vi "single fit V5cpp.vi"(0 "single fit parameters":T11={"number of 2D grid points"=300, "# of points in pond"=339, "# of points in window"=10919, "decimation threshold"=1, "normalization factor"=0.029014793, "pond scale factor "=3.0, "normalized z"=[], "decimated z"=[], "decimated omega"=[], "omega in window"=[], "z in window"=[], "data center"=3.0+0.0i, "inverse"=[], "linear "=[], "omega around"=[], "phase around center"=[], "fit for phase around senter "=[], "three points"={[], []}, "max omega"=0.029014793, "min omega"=0.029014793, "dz/domega"=[]}, 1 "plot what":enum16{"plot", "dont plot", "a"}(ring), 2 "find fit action":T8=enum."bbb", 3 "cursor bracket: fragment  ref":refnum<vi>, 5 "omega map parameters":T10={"map method"=enum."less trivial", "2:window factor"=1, "left"=3.0, "right"=3.0, "omega"=3.0, "gamma"=3.0, "theta0"=3.0, "use points"=enum."decimated", "z(inf) method"=enum."median"}, 7 "parameters: wavepacket":T4={"R"=0.5, "wave number"=9.317073170731707, "delta k"=8.0, "radii vector"=[-1.5, -1.4361702127659575, -1.372340425531915, -1.3085106382978724, -1.2446808510638299, -1.1808510638297873, -1.1170212765957448, -1.0531914893617023, -0.9893617021276596, -0.9255319148936171, -0.8617021276595745, -0.797872340425532, -0.7340425531914894, -0.6702127659574468, -0.6063829787234043, -0.5425531914893618, -0.47872340425531923, -0.4148936170212767, -0.35106382978723416, -0.2872340425531916, -0.2234042553191491, -0.15957446808510656, -0.09574468085106402, -0.03191489361702149, 0.03191489361702127, 0.0957446808510638, 0.15957446808510634, 0.22340425531914887, 0.2872340425531914, 0.35106382978723394, 0.4148936170212765, 0.478723404255319, 0.5425531914893615, 0.6063829787234041, 0.6702127659574466, 0.7340425531914891, 0.7978723404255317, 0.8617021276595742, 0.9255319148936167, 0.9893617021276593, 1.0531914893617018, 1.1170212765957444, 1.1808510638297869, 1.2446808510638294, 1.308510638297872, 1.3723404255319145, 1.436170212765957], "radial section"=[-0.0004435445083409722-0.0006849119769038184i, -0.0019041504025470312+0.00048506615579312746i, -0.00033819317362592454+0.00445256884703147i, 0.008816469374270853+0.0037385059601190047i, 0.012871051762105094-0.014489928742809924i, -0.018368300887416027-0.03213667871181133i, -0.06546452421830008+0.012862287260149104i, -0.014850036489490822+0.11250194158627941i, 0.16349796399613198+0.08029027224632529i, 0.19438455385148304-0.19581588584379236i, -0.1764517694229995-0.3527505964833319i, -0.5269831636950821+0.07349813170268539i, -0.12571385568454752+0.6656158756342778i, 0.7094879059571741+0.3986438774133789i, 0.6853115356988965-0.6177994674685856i, -0.39205198313530026-0.9060192033187687i, -0.9933425353192824+0.08278273424671147i, -0.22770617853759392+0.9220982637950581i, 0.720265950295077+0.4589746661280373i, 0.564369978321562-0.45471185099562045i, -0.20063123992670956-0.5446207511436068i, -0.438459632746935+0.012155082564416607i, -0.0917074180027409+0.299079584121901i, 0.17101533661135507+0.12280738192151135i, 0.17101533661135532+0.1228073819215104i, -0.0917074180027395+0.299079584121901i, -0.4384596327469345+0.01215508256441854i, -0.2006312399267118-0.5446207511436055i, 0.5643699783215596-0.4547118509956226i, 0.7202659502950789+0.45897466612803384i, -0.22770617853759056+0.9220982637950585i, -0.9933425353192818+0.08278273424671675i, -0.3920519831353035-0.9060192033187675i, 0.6853115356988935-0.6177994674685894i, 0.7094879059571758+0.3986438774133766i, -0.12571385568454407+0.665615875634279i, -0.5269831636950825+0.0734981317026883i, -0.17645176942300106-0.3527505964833319i, 0.19438455385148207-0.19581588584379414i, 0.16349796399613292+0.0802902722463243i, -0.014850036489490074+0.11250194158627992i, -0.06546452421830022+0.012862287260149614i, -0.018368300887416446-0.032136678711811265i, 0.012871051762104992-0.014489928742810118i, 0.008816469374270927+0.0037385059601189627i, -0.0003381931736258947+0.004452568847031496i, -0.0019041504025470377+0.00048506615579315077i], "wave vector"=19.513632417419526, "wavepacket is"=TRUE} {"delta k" format="%#_3f"; "wave number" format="%#_3f"; "R" format="%#_3f"}, 9 "parameters: complex fit":T3={"main VI path"=path "", "scale factor"=3.0, "# of grid points"=200, "parameters: wavepacket"={"R"=0.5, "wave number"=22.0, "delta k"=7.0, "radii vector"=[], "radial section"=[], "wave vector"=22.0, "wavepacket is"=TRUE}, "span"=0.27789, "interference ?"=enum."cp z center", "filter method"=enum."three"} {"span" min=0.0 max=0.5 step=1e-05 scale=0.0001..0.5 scale format="%#_5f"; "parameters: wavepacket"."delta k" format="%#_3f"; "parameters: wavepacket"."wave number" format="%#_3f"; "parameters: wavepacket"."R" format="%#_3f"}, 11 "input":cdb, 13 "plots: filter related":T6) -> (4 "single fit parameters out":T11={"number of 2D grid points"=300, "# of points in pond"=339, "# of points in window"=10919, "decimation threshold"=1, "normalization factor"=0.029014793, "pond scale factor "=3.0, "normalized z"=[], "decimated z"=[], "decimated omega"=[], "omega in window"=[], "z in window"=[], "data center"=3.0+0.0i, "inverse"=[], "linear "=[], "omega around"=[], "phase around center"=[], "fit for phase around senter "=[], "three points"={[], []}, "max omega"=0.029014793, "min omega"=0.029014793, "dz/domega"=[]}, 6 "omega map parameters out":T10={"map method"=enum."less trivial", "2:window factor"=1, "left"=3.0, "right"=3.0, "omega"=3.0, "gamma"=3.0, "theta0"=3.0, "use points"=enum."decimated", "z(inf) method"=enum."median"}, 8 "parameters: wavepacket  out":T4={"R"=0.5, "wave number"=9.317073170731707, "delta k"=8.0, "radii vector"=[-1.5, -1.4361702127659575, -1.372340425531915, -1.3085106382978724, -1.2446808510638299, -1.1808510638297873, -1.1170212765957448, -1.0531914893617023, -0.9893617021276596, -0.9255319148936171, -0.8617021276595745, -0.797872340425532, -0.7340425531914894, -0.6702127659574468, -0.6063829787234043, -0.5425531914893618, -0.47872340425531923, -0.4148936170212767, -0.35106382978723416, -0.2872340425531916, -0.2234042553191491, -0.15957446808510656, -0.09574468085106402, -0.03191489361702149, 0.03191489361702127, 0.0957446808510638, 0.15957446808510634, 0.22340425531914887, 0.2872340425531914, 0.35106382978723394, 0.4148936170212765, 0.478723404255319, 0.5425531914893615, 0.6063829787234041, 0.6702127659574466, 0.7340425531914891, 0.7978723404255317, 0.8617021276595742, 0.9255319148936167, 0.9893617021276593, 1.0531914893617018, 1.1170212765957444, 1.1808510638297869, 1.2446808510638294, 1.308510638297872, 1.3723404255319145, 1.436170212765957], "radial section"=[-0.0004435445083409722-0.0006849119769038184i, -0.0019041504025470312+0.00048506615579312746i, -0.00033819317362592454+0.00445256884703147i, 0.008816469374270853+0.0037385059601190047i, 0.012871051762105094-0.014489928742809924i, -0.018368300887416027-0.03213667871181133i, -0.06546452421830008+0.012862287260149104i, -0.014850036489490822+0.11250194158627941i, 0.16349796399613198+0.08029027224632529i, 0.19438455385148304-0.19581588584379236i, -0.1764517694229995-0.3527505964833319i, -0.5269831636950821+0.07349813170268539i, -0.12571385568454752+0.6656158756342778i, 0.7094879059571741+0.3986438774133789i, 0.6853115356988965-0.6177994674685856i, -0.39205198313530026-0.9060192033187687i, -0.9933425353192824+0.08278273424671147i, -0.22770617853759392+0.9220982637950581i, 0.720265950295077+0.4589746661280373i, 0.564369978321562-0.45471185099562045i, -0.20063123992670956-0.5446207511436068i, -0.438459632746935+0.012155082564416607i, -0.0917074180027409+0.299079584121901i, 0.17101533661135507+0.12280738192151135i, 0.17101533661135532+0.1228073819215104i, -0.0917074180027395+0.299079584121901i, -0.4384596327469345+0.01215508256441854i, -0.2006312399267118-0.5446207511436055i, 0.5643699783215596-0.4547118509956226i, 0.7202659502950789+0.45897466612803384i, -0.22770617853759056+0.9220982637950585i, -0.9933425353192818+0.08278273424671675i, -0.3920519831353035-0.9060192033187675i, 0.6853115356988935-0.6177994674685894i, 0.7094879059571758+0.3986438774133766i, -0.12571385568454407+0.665615875634279i, -0.5269831636950825+0.0734981317026883i, -0.17645176942300106-0.3527505964833319i, 0.19438455385148207-0.19581588584379414i, 0.16349796399613292+0.0802902722463243i, -0.014850036489490074+0.11250194158627992i, -0.06546452421830022+0.012862287260149614i, -0.018368300887416446-0.032136678711811265i, 0.012871051762104992-0.014489928742810118i, 0.008816469374270927+0.0037385059601189627i, -0.0003381931736258947+0.004452568847031496i, -0.0019041504025470377+0.00048506615579315077i], "wave vector"=19.513632417419526, "wavepacket is"=TRUE} {"delta k" format="%#_3f"; "wave number" format="%#_3f"; "R" format="%#_3f"}, 14 "complex region out":T7={"max re"=1.1965102077412717, "min re"=-1.8034897922587283, "max im"=1.1920568931854867, "min im"=-1.636084117505164, "delta re"=3.0, "delta im"=2.8281410106906506, "center re"=-0.3034897922587282, "delta  z"=3.0+2.8281410106906506i, "center im"=-0.2220136121598386, "center z"=-0.3034897922587282+2.8281410106906506i, "d im"=0.0, "d re"=0.0, "d z"=0.0+0.0i}, 15 "lorentzian out":T1={"A (VHz)"=-1.0311345636926572, "ω (Hz)"=-1.0311345636926572, "Γ (Hz)"=-1.0311345636926572, "φ (rad)"=-1.0311345636926572, "Q"=-1.0311345636926572, "Norm  Ampl"=-1.0311345636926572, "z∞ (V)"=-1.0311345636926572+0.0i, "4corners"={"z (-pi/2)"=-1.0311345636926572+0.5736824521422934i, "z(inf)"=-0.5200164984937075+1.0975277942502903i, "z (pi/2)"=-1.0311345636926572+0.5736824521422934i, "z center"=-0.5136528600391839+0.580046090596817i, "z(0)"=-0.5200164984937075+1.0975277942502903i, "radius"=-1.0311345636926572}} {"z∞ (V)" format="%#_4p"; "Q" format="%#_4p"; "φ (rad)" format="%#_3p"; "Γ (Hz)" format="%#_5p"; "ω (Hz)" format="%#_9p"; "A (VHz)" format="%#_3p"})   [LabVIEW 2021]
uses:
  circle corners.ctl
  lorentzian.ctl
  find peak action.ctl
  stack action -- control.ctl
  cursor window action.ctl
  circledll.dll
  complex region.ctl
  single fit parameters.ctl
  omega map parameters.ctl
  cursor winow.ctl
  wavepacket.ctl
  plot refs -- filter related.ctl
  filter method control.ctl
  peak -- parameters -- complex fit.ctl
panel:
  out "counter_out":i32
  out "# points in window":dbl
  out "good lorentzian":T1={"A (VHz)"=-1.0311345636926572, "ω (Hz)"=-1.0311345636926572, "Γ (Hz)"=-1.0311345636926572, "φ (rad)"=-1.0311345636926572, "Q"=-1.0311345636926572, "Norm  Ampl"=-1.0311345636926572, "z∞ (V)"=-1.0311345636926572+0.0i, "4corners"={"z (-pi/2)"=-1.0311345636926572+0.5736824521422934i, "z(inf)"=-0.5200164984937075+1.0975277942502903i, "z (pi/2)"=-1.0311345636926572+0.5736824521422934i, "z center"=-0.5136528600391839+0.580046090596817i, "z(0)"=-0.5200164984937075+1.0975277942502903i, "radius"=-1.0311345636926572}} {"z∞ (V)" format="%#_4p"; "Q" format="%#_4p"; "φ (rad)" format="%#_3p"; "Γ (Hz)" format="%#_5p"; "ω (Hz)" format="%#_9p"; "A (VHz)" format="%#_3p"}
  out "cp lorentzian":T1={"A (VHz)"=-1.0311345636926572, "ω (Hz)"=-1.0311345636926572, "Γ (Hz)"=-1.0311345636926572, "φ (rad)"=-1.0311345636926572, "Q"=-1.0311345636926572, "Norm  Ampl"=-1.0311345636926572, "z∞ (V)"=-1.0311345636926572+0.0i, "4corners"={"z (-pi/2)"=-1.0311345636926572+0.5736824521422934i, "z(inf)"=-0.5200164984937075+1.0975277942502903i, "z (pi/2)"=-1.0311345636926572+0.5736824521422934i, "z center"=-0.5136528600391839+0.580046090596817i, "z(0)"=-0.5200164984937075+1.0975277942502903i, "radius"=-1.0311345636926572}} {"z∞ (V)" format="%#_4p"; "Q" format="%#_4p"; "φ (rad)" format="%#_3p"; "Γ (Hz)" format="%#_5p"; "ω (Hz)" format="%#_9p"; "A (VHz)" format="%#_3p"}
  out "pm lorentzian":T1={"A (VHz)"=-1.0311345636926572, "ω (Hz)"=-1.0311345636926572, "Γ (Hz)"=-1.0311345636926572, "φ (rad)"=-1.0311345636926572, "Q"=-1.0311345636926572, "Norm  Ampl"=-1.0311345636926572, "z∞ (V)"=-1.0311345636926572+0.0i, "4corners"={"z (-pi/2)"=-1.0311345636926572+0.5736824521422934i, "z(inf)"=-0.5200164984937075+1.0975277942502903i, "z (pi/2)"=-1.0311345636926572+0.5736824521422934i, "z center"=-0.5136528600391839+0.580046090596817i, "z(0)"=-0.5200164984937075+1.0975277942502903i, "radius"=-1.0311345636926572}} {"z∞ (V)" format="%#_4p"; "Q" format="%#_4p"; "φ (rad)" format="%#_3p"; "Γ (Hz)" format="%#_5p"; "ω (Hz)" format="%#_9p"; "A (VHz)" format="%#_3p"}
  in  "window factor - max":i32=10
  in  "window factor - min":i32=10
  out "bb 2":dbl
  out "directed sigma 2":dbl
  out "right 2":cdb
  out "left 2":cdb
  out "Numeric 2":i32
  in  "averaging -- win 2":dbl=1.3
  in  "averaging -- span 2":dbl=0.2
  in  "averaging -- # points 2":i32=30
  in  "averaging -- # points":i32=30
  in  "averaging -- span":dbl=0.2
  in  "averaging -- win":dbl=1.3
  out "Numeric":i32
  out "left":cdb
  out "right":cdb
  out "directed sigma":dbl
  out "bb":dbl
  in  "complex region":T7={"max re"=1.1965102077412717, "min re"=-1.8034897922587283, "max im"=1.1920568931854867, "min im"=-1.636084117505164, "delta re"=3.0, "delta im"=2.8281410106906506, "center re"=-0.3034897922587282, "delta  z"=3.0+2.8281410106906506i, "center im"=-0.2220136121598386, "center z"=-0.3034897922587282+2.8281410106906506i, "d im"=0.0, "d re"=0.0, "d z"=0.0+0.0i}
  in  "cursor bracket in":T9={"left"=2044.0881763527054, "right "=2126.7657992565055, "center"=2085.4269878046052, "window"=82.67762290380006, "cursors"=[], "relative"=0, "absolute"=0, "fixed vertical offset"=2421.6740576496672, "vertical offset"=2421.6740576496672, "skew"=2421.6740576496672, "default window frac"=2421.6740576496672, "kind"=enum."fancy", "skew.left"=2.0, "skew.right"=0.0, "Plot ref"=refnum, "wing order"=enum."back"}
  in  "factor":dbl=7.0
  in  "pond":cdb[][](array[numeric])
  in  "wave packet":cdb[][](array[numeric])
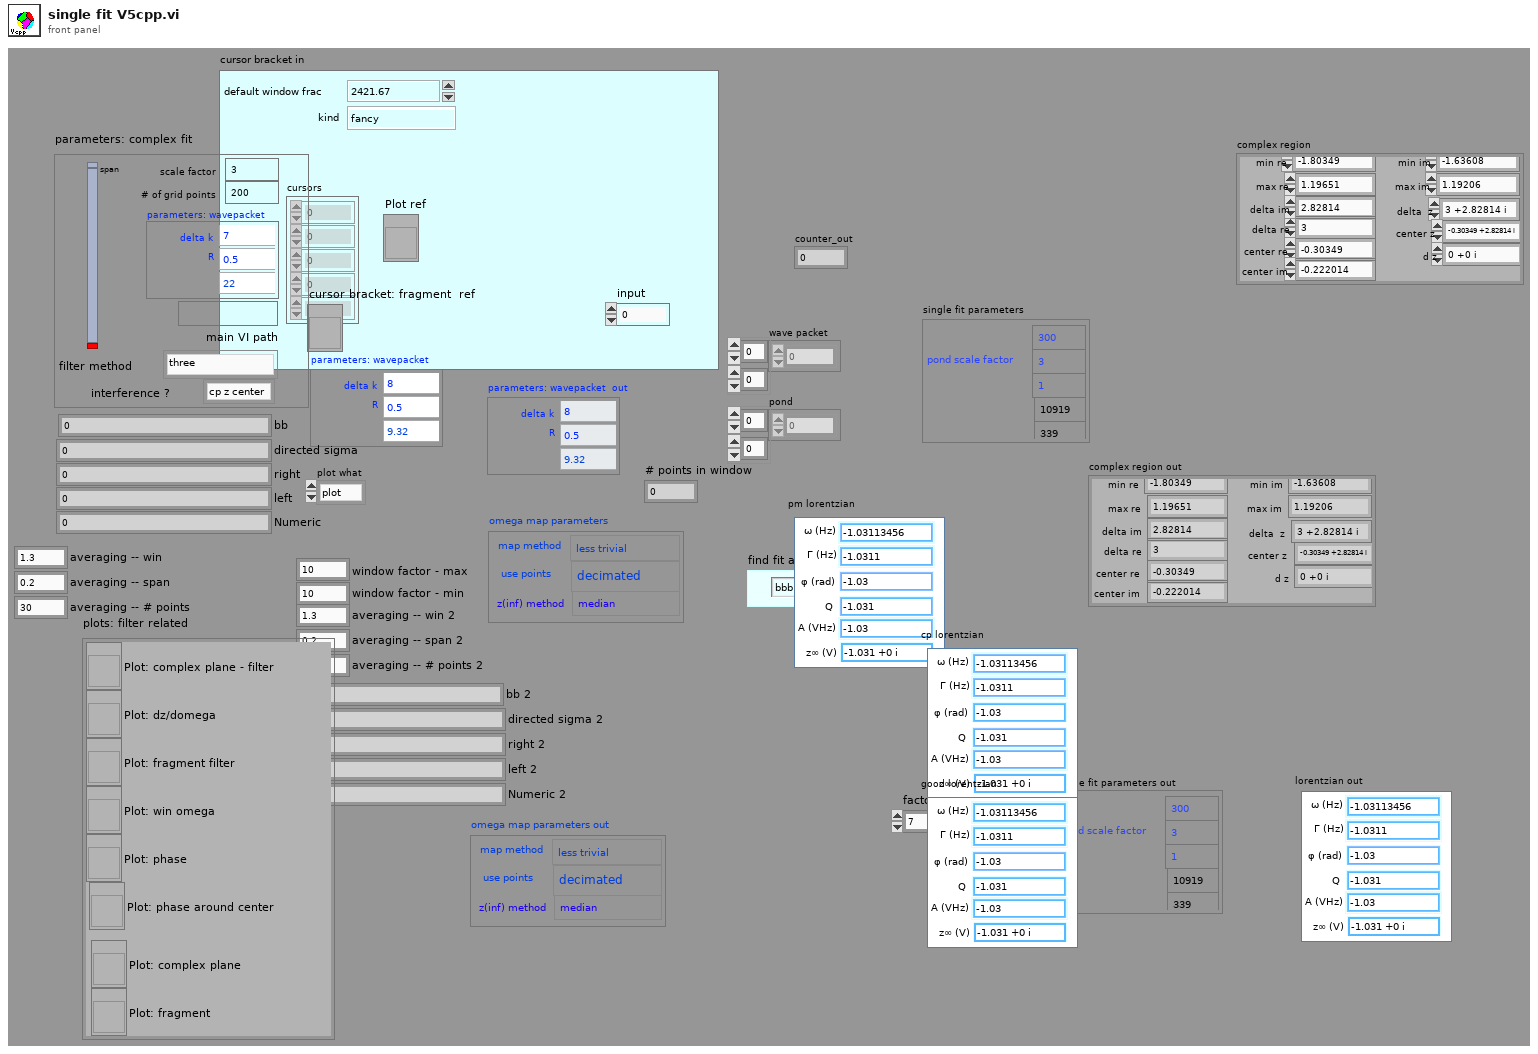
[diagram p1: front panel]
types:
  T1 = typedef "lorentzian.ctl" = cluster{"A (VHz)":dbl, "ω (Hz)":dbl, "Γ (Hz)":dbl, "φ (rad)":dbl, "Q":dbl, "Norm  Ampl":dbl, "z∞ (V)":cdb, "4corners":T2}
  T2 = typedef "circle corners.ctl" = cluster{"z (-pi/2)":cdb, "z(inf)":cdb, "z (pi/2)":cdb, "z center":cdb, "z(0)":cdb, "radius":dbl}
  T3 = typedef "peak -- parameters -- complex fit.ctl" = cluster{"main VI path":path, "scale factor":dbl, "# of grid points":i32, "parameters: wavepacket":T4, "span":dbl, "interference ?":enum16{"cp z center", "pm zcenter", "fancy"}, "filter method":T5}
  T4 = typedef "wavepacket.ctl" = cluster{"R":dbl, "wave number":dbl, "delta k":dbl, "radii vector":dbl[], "radial section":cdb[], "wave vector":dbl, "wavepacket is":bool}
  T5 = typedef "filter method control.ctl" = enum16{"four", "five", "one", "two", "three", "zero", "minus one", "minus two"}
  T6 = typedef "plot refs -- filter related.ctl" = cluster{"Plot: complex plane - filter":refnum<vi>, "Plot: dz/domega":refnum<vi>, "Plot: fragment filter":refnum<vi>, "Plot: win omega":refnum<vi>, "Plot: phase":refnum<vi>, "Plot: phase around center":refnum<vi>, "Plot: complex plane":refnum<vi>, "Plot: fragment":refnum<vi>}
  T7 = typedef "complex region.ctl" = cluster{"max re":dbl, "min re":dbl, "max im":dbl, "min im":dbl, "delta re":dbl, "delta im":dbl, "center re":dbl, "delta  z":cdb, "center im":dbl, "center z":cdb, "d im":dbl, "d re":dbl, "d z":cdb}
  T8 = typedef "find peak action.ctl" = enum16{"empty", "-find center", "-mapping", "fit", "-shake it one", "bbb", "-update pond", "move z(center)", "move z(inf)", "update pond", "fancy fit one", "fragment window moves", "-shake it two", "fancy fit two", "pm fit"}
  T9 = typedef "cursor winow.ctl" = cluster{"left":dbl, "right ":dbl, "center":dbl, "window":dbl, "cursors":i32[], "relative":i32, "absolute":i32, "fixed vertical offset":dbl, "vertical offset":dbl, "skew":dbl, "default window frac":dbl, "kind":enum16{"symmetric", "skewed", "fancy"}, "skew.left":dbl, "skew.right":dbl, "Plot ref":refnum<vi>, "wing order":enum16{"forw", "back"}}
  T10 = typedef "omega map parameters.ctl" = cluster{"map method":enum16{"simple", "less trivial", "around center", "geometry"}, "2:window factor":i32, "left":dbl, "right":dbl, "omega":dbl, "gamma":dbl, "theta0":dbl, "use points":enum16{"all in window", "decimated"}, "z(inf) method":enum16{"median", "method 2", "histogram"}}
  T11 = typedef "single fit parameters.ctl" = cluster{"number of 2D grid points":i32, "# of points in pond":i32, "# of points in window":i32, "decimation threshold":i32, "normalization factor":dbl, "pond scale factor ":dbl, "normalized z":cdb[], "decimated z":cdb[], "decimated omega":dbl[], "omega in window":dbl[], "z in window":cdb[], "data center":cdb, "inverse":cdb[], "linear ":cdb[], "omega around":dbl[], "phase around center":dbl[], "fit for phase around senter ":dbl[], "three points":cluster{dbl[], dbl[]}, "max omega":dbl, "min omega":dbl, "dz/domega":cdb[]}
  T12 = cluster{"cursor bracket: fragment  ref":refnum<vi>, "main VI path":path, "fancy fit":cluster{"z(center)":cdb, "center":dbl, "window":dbl, "omega ave":dbl, "gamma ave":dbl, "shakeit counter":i32, "current center":dbl, "current window":dbl}}
  T13 = typedef "stack action -- control.ctl" = enum16{"push", "pop", "check", "init"}
  T14 = typedef "cursor window action.ctl" = enum16{"balance", "h. offset change", "cursor moves", "change center", "change window", "init", "check", "reset", "set y to middle", "idle", "-write all Y", "-write left.X", "-write center.X", "-write right.X", "-write all X", "-change center", "-change window", "-change skew", "-read cursor 2", "-read cursor 1", "-read cursor 0", "-read all cursors", "-reset", "-read plot scale", "-set y to middle", "-Q: center.Y is visible", "-Q: window is visible", "-parse center.Y", "-right left from center", "-left move", "-right move", "-set center.Y", "-empty", "-set cursors to default", "-check", "-write center.Y", "-copy cursor 1", "-copy cursor 0", "-copy cursor 2", "move right", "move left", "shrink", "broaden", "skew up", "skew down", "-write plot scale", "zoom X", "change cen&win", "zoom to all data", "color--red", "color--green", "color--yellow", "read", "zoom out", "zoom in", "slide right", "slide left", "set range aspect ratio to 1", "move to window range", "--move to window range"}
  T15 = typedef "comparison control.ctl" = enum16{"not a number", "above", "in range", "below"}
  T16 = cluster{"left":dbl, "right ":dbl, "center":dbl, "window":dbl, "cursors":i32[], "relative":i32, "absolute":i32, "fixed vertical offset":dbl, "vertical offset":dbl, "skew":dbl, "default window frac":dbl, "kind":enum16{"symmetric", "skewed", "fancy"}, "skew.left":dbl, "skew.right":dbl, "Plot ref":refnum<vi>, "wing order":enum16{"forw", "back"}}
  T17 = enum16{"replace z(center) -- keepin z(inf) the same", "replace z(inf)  -- keeping z(center) the same"}
  T18 = typedef "tale of three indices -- int -- control.ctl" = cluster{"left":i32, "center":i32, "right":i32, "right most":i32, "left most":i32, "window":i32, "max win factor":i32, "max win":i32, "min win":i32}
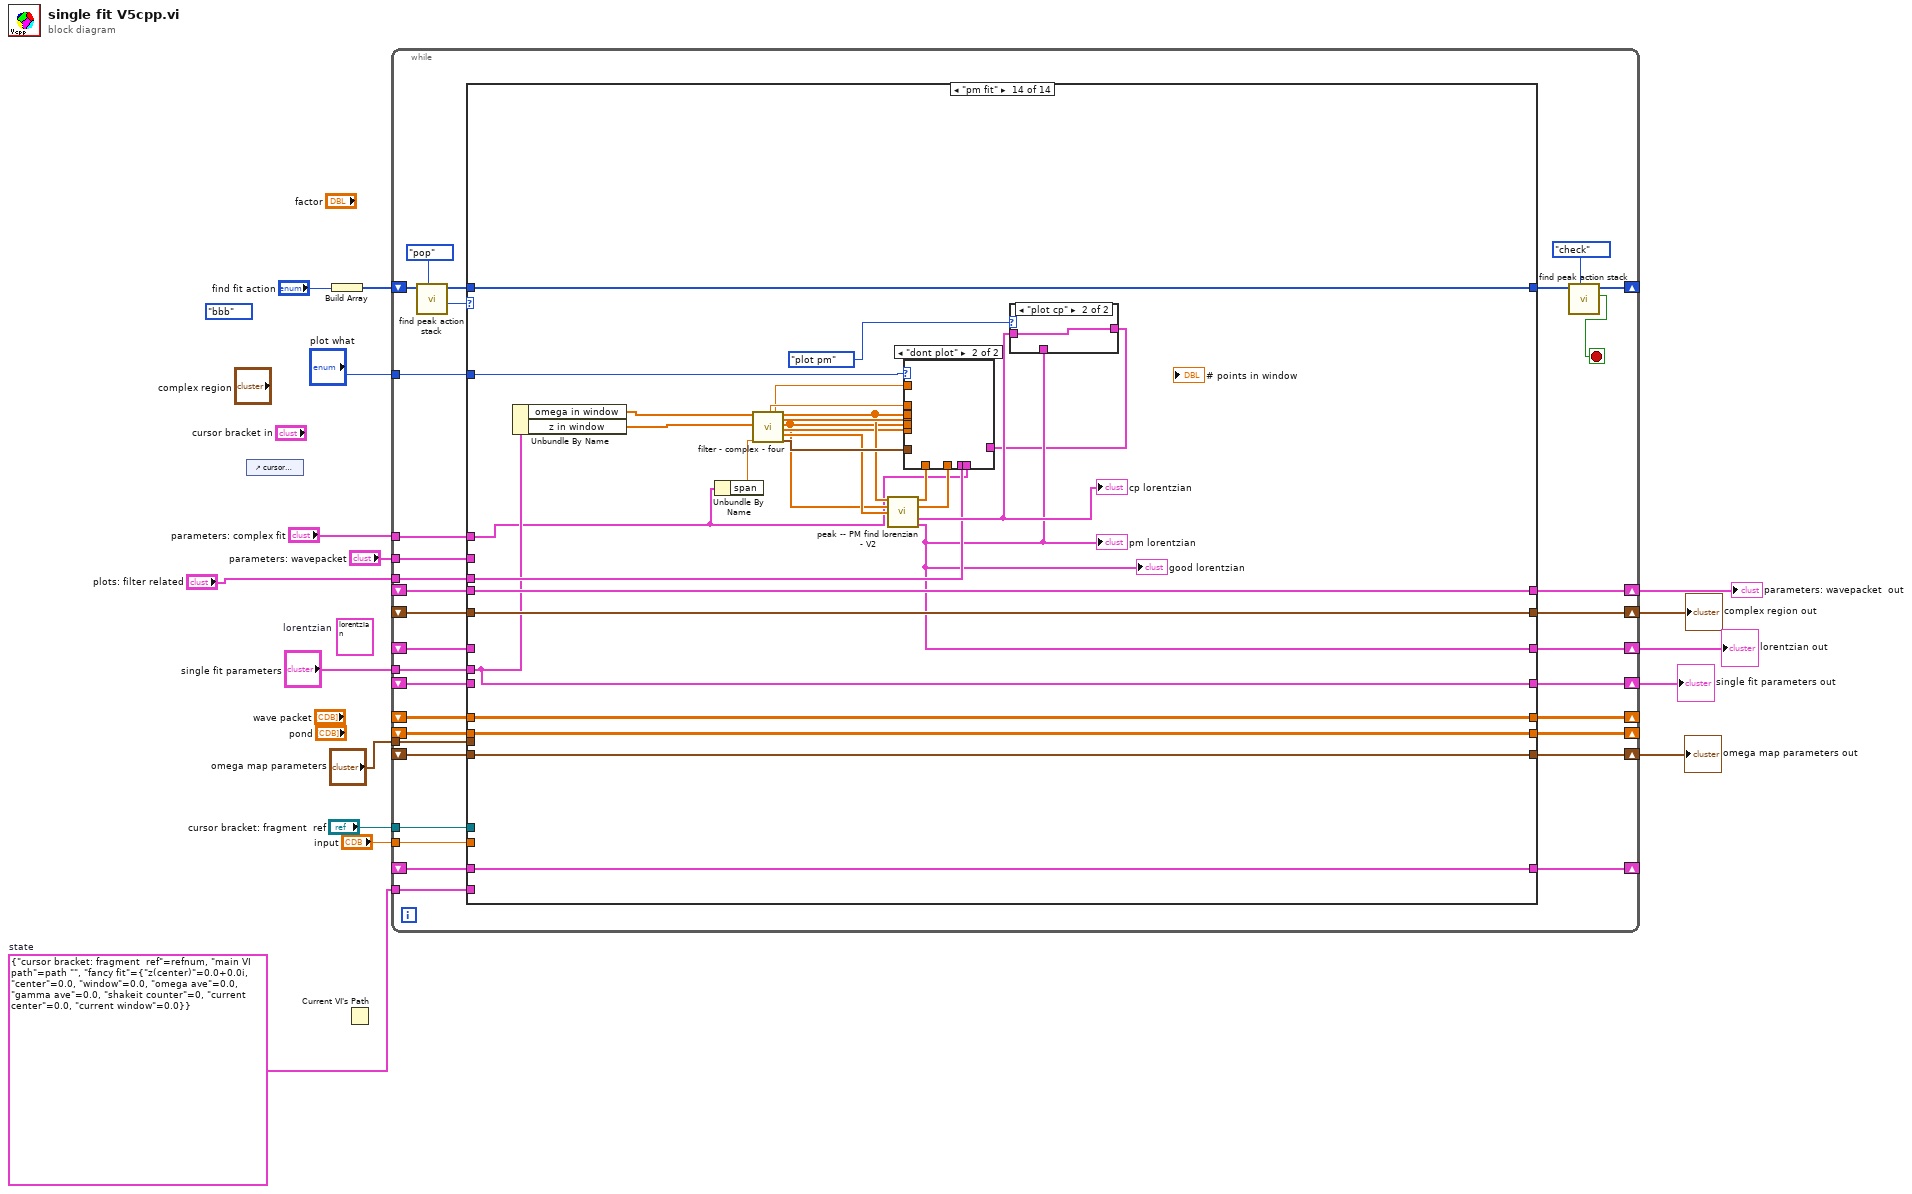
[diagram p0: block diagram]
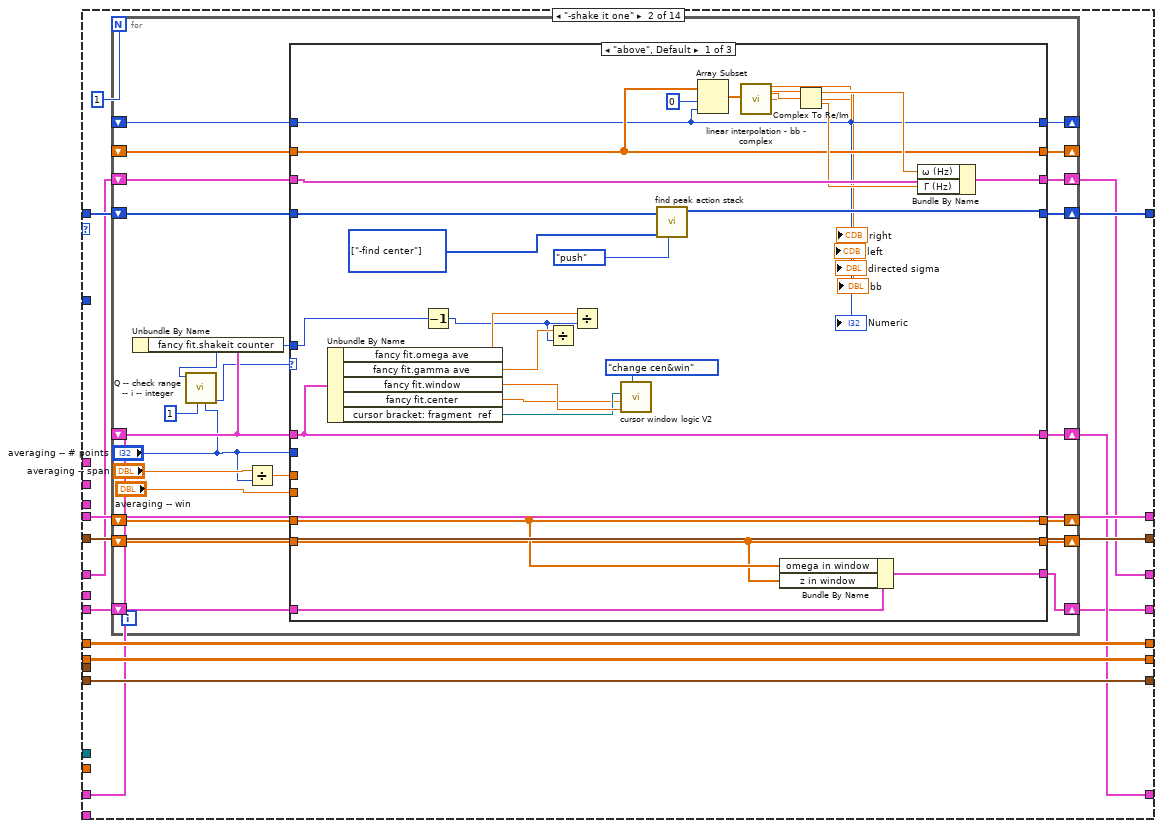
[diagram p3: hidden frame]
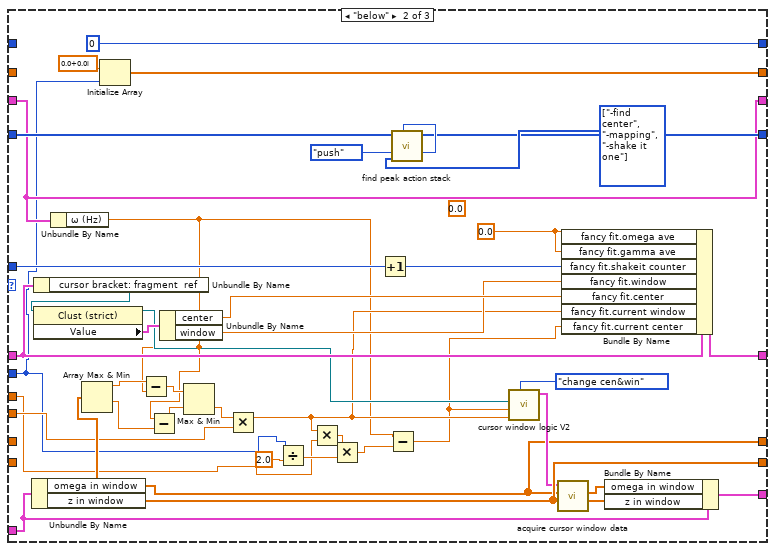
[diagram p4: hidden frame]
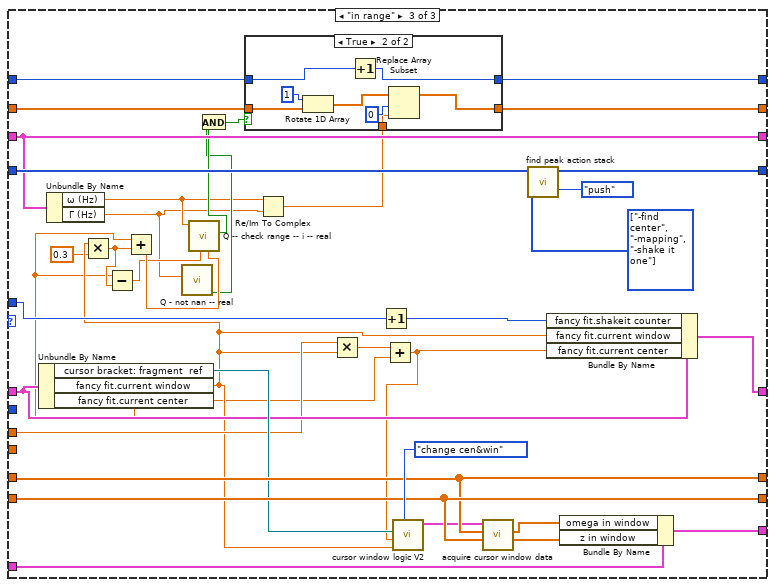
[diagram p5: hidden frame]
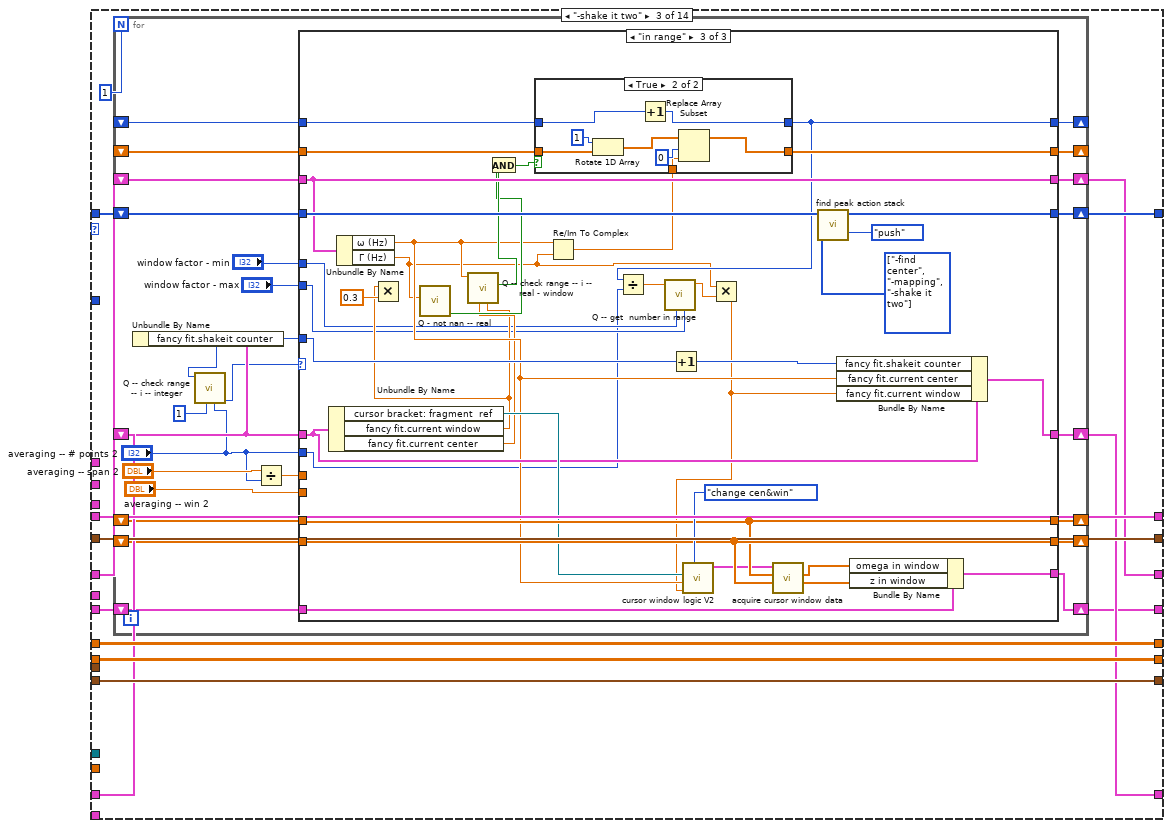
[diagram p7: hidden frame]
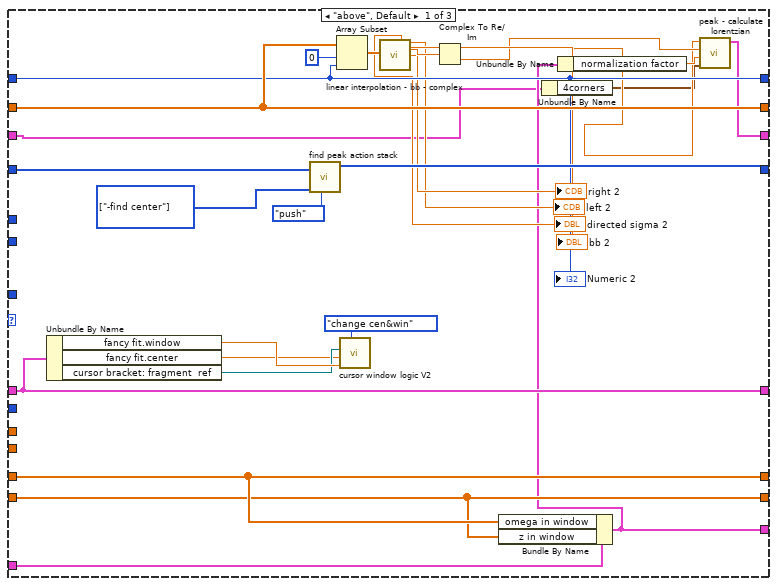
[diagram p8: hidden frame]
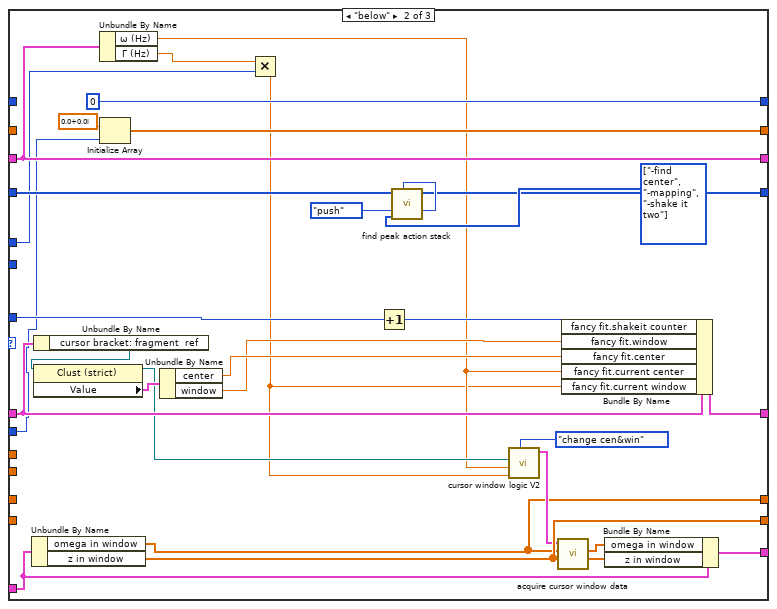
[diagram p9: hidden frame]
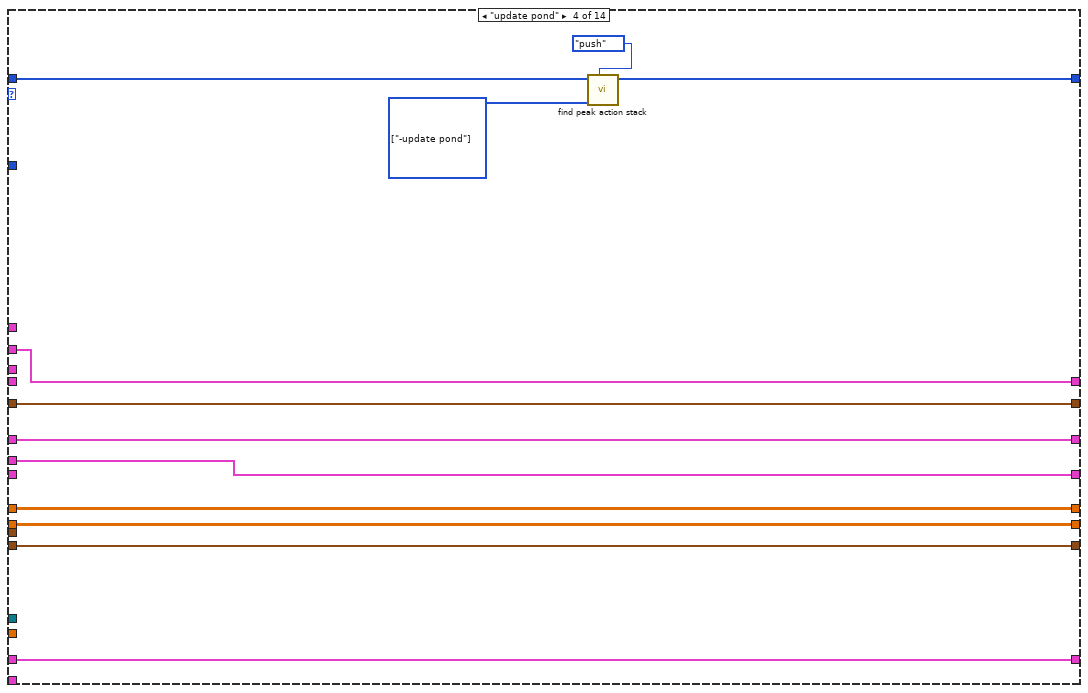
[diagram p11: hidden frame]
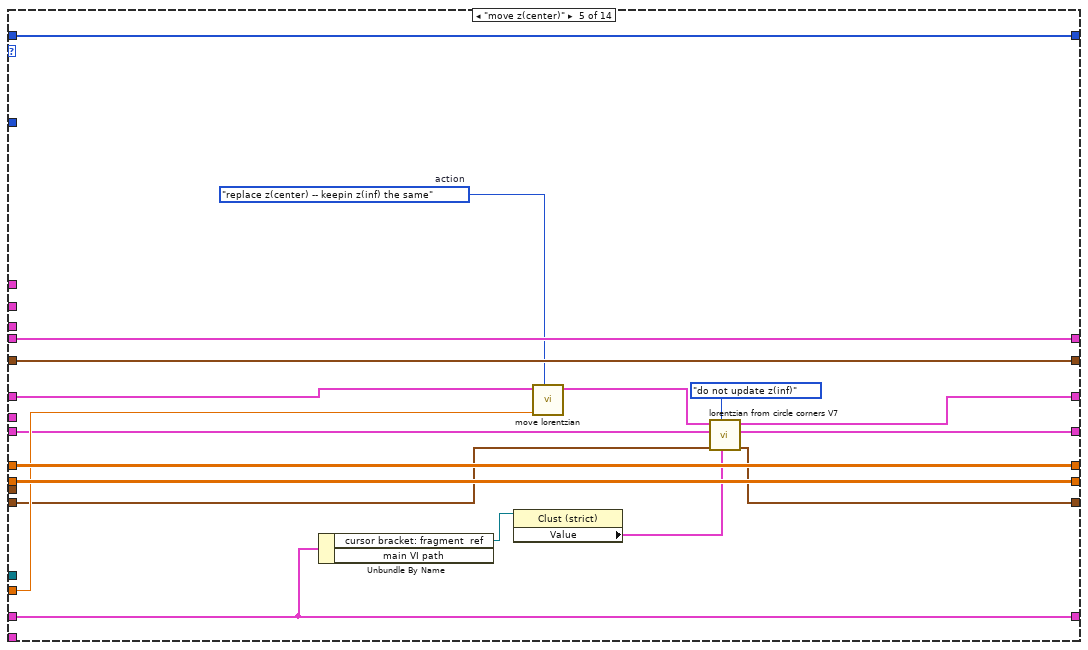
[diagram p12: hidden frame]
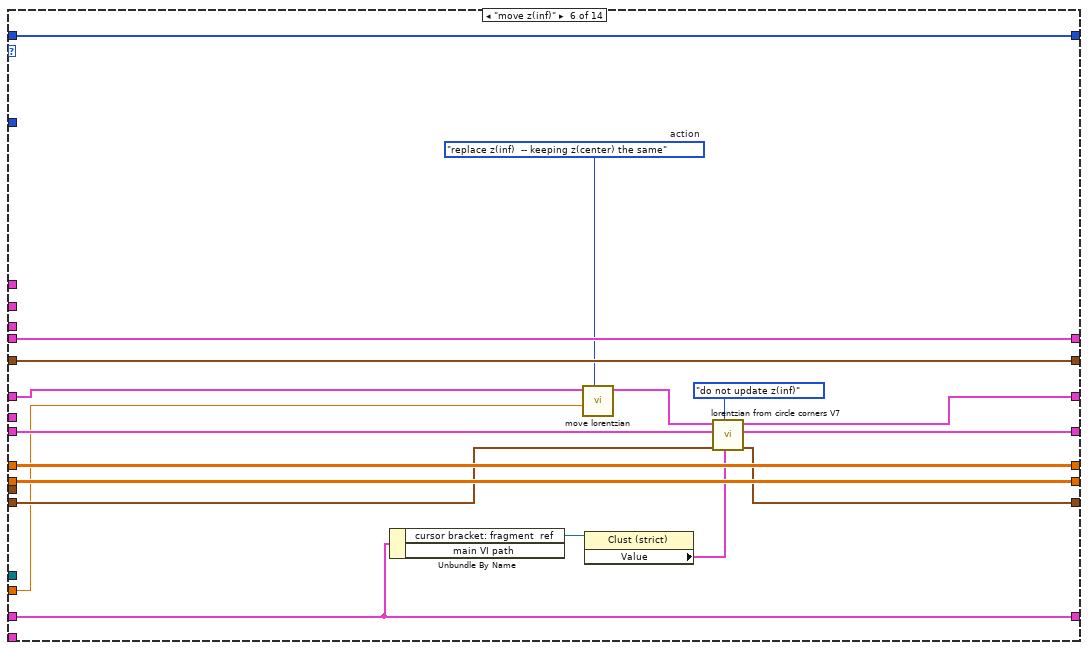
[diagram p13: hidden frame]
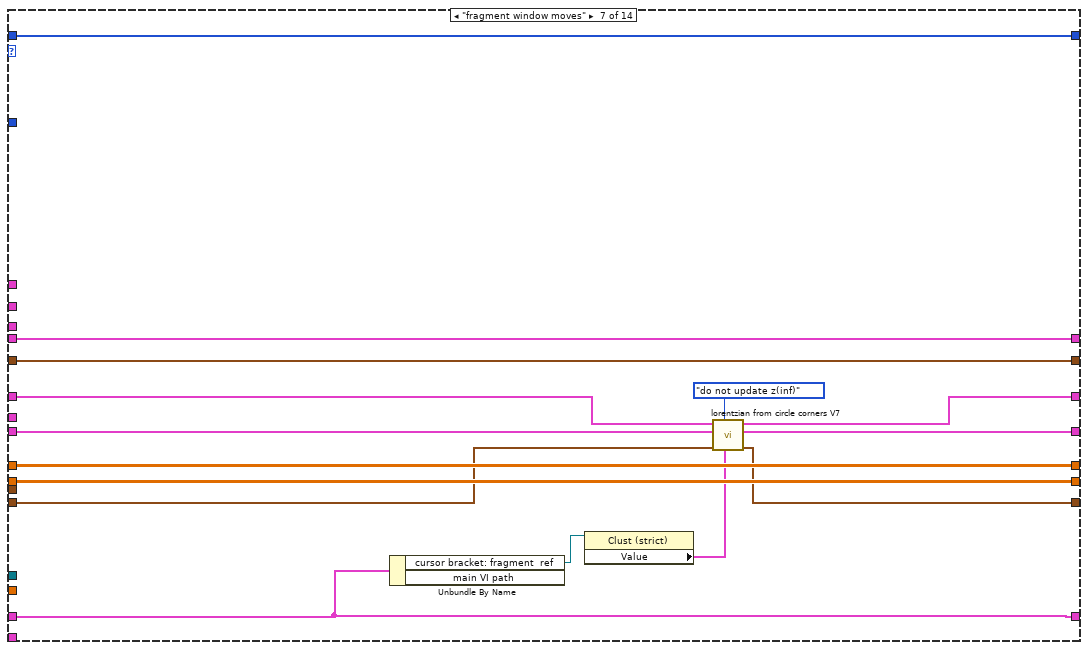
[diagram p14: hidden frame]
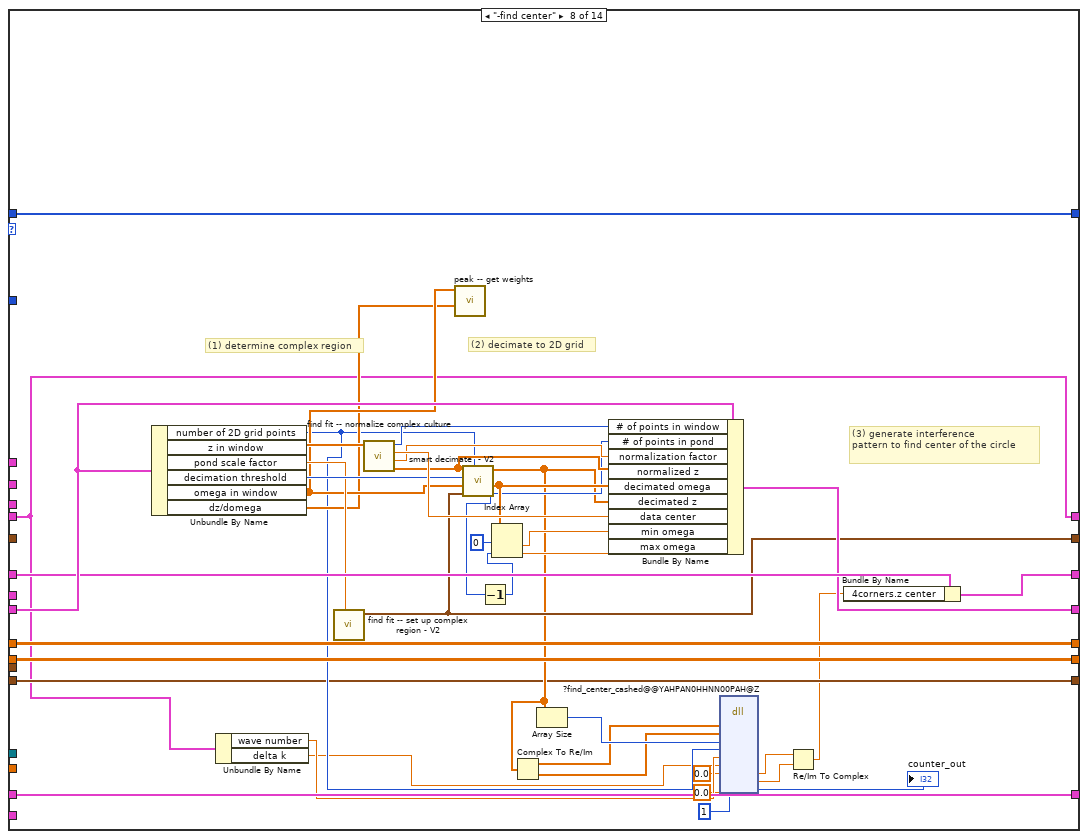
[diagram p15: hidden frame]
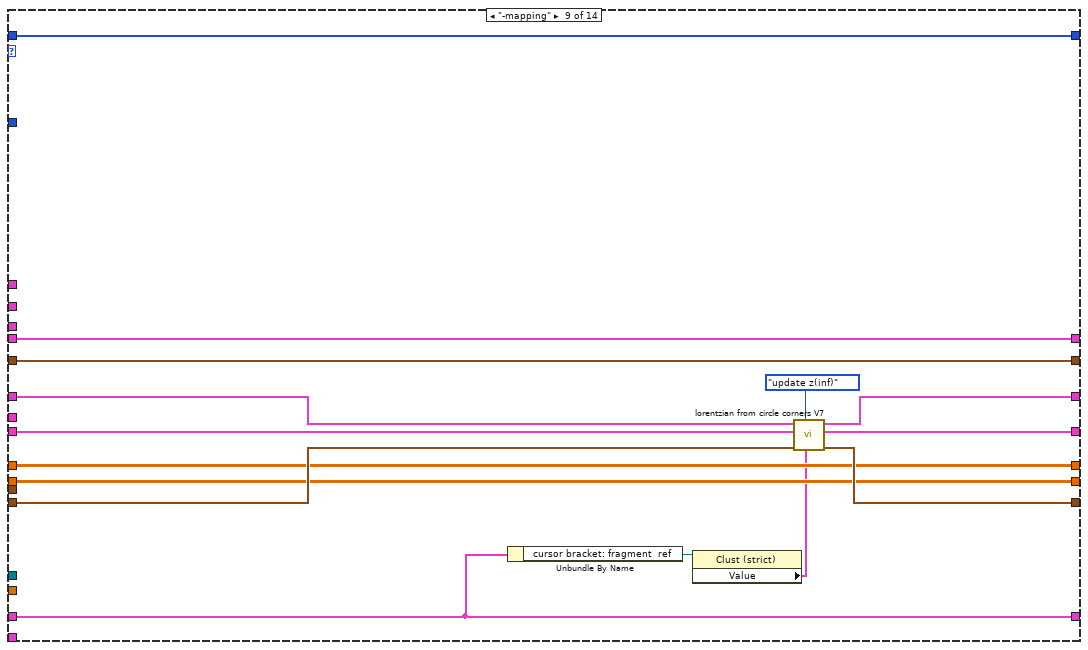
[diagram p16: hidden frame]
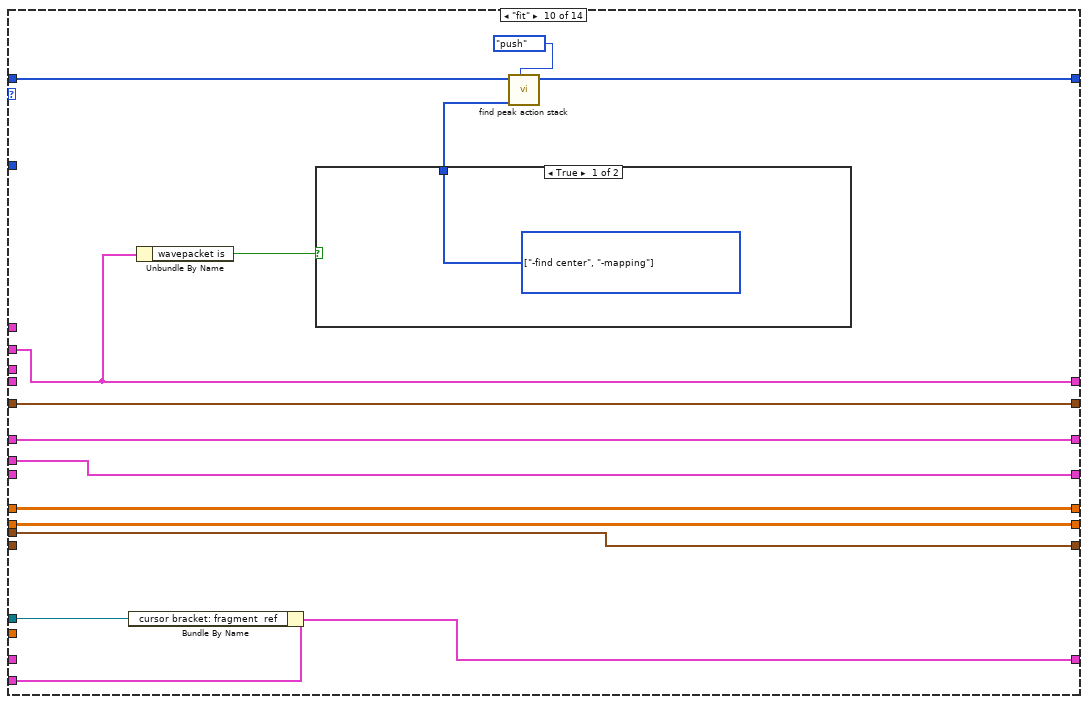
[diagram p17: hidden frame]
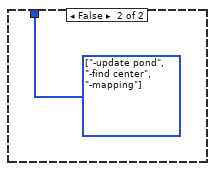
[diagram p18: hidden frame]
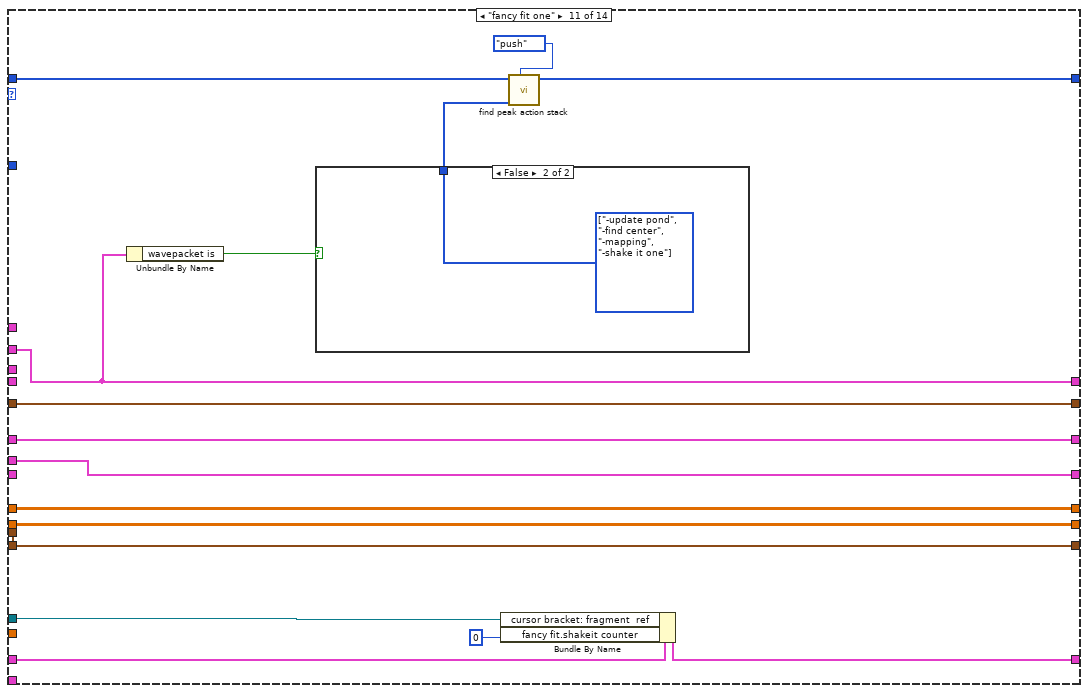
[diagram p19: hidden frame]
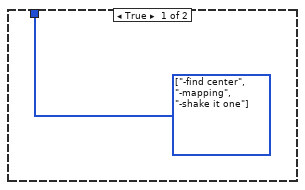
[diagram p20: hidden frame]
diagram:
  w4 = T12 {"cursor bracket: fragment  ref"=refnum, "main VI path"=path "", "fancy fit"={"z(center)"=0.0+0.0i, "center"=0.0, "window"=0.0, "omega ave"=0.0, "gamma ave"=0.0, "shakeit counter"=0, "current center"=0.0, "current window"=0.0}}  # state
  (unwired) find_peak_action."bbb" ("find fit action")
  (unwired) T1 {"A (VHz)"=-1.0311345636926572, "ω (Hz)"=-1.0311345636926572, "Γ (Hz)"=-1.0311345636926572, "φ (rad)"=-1.0311345636926572, "Q"=-1.0311345636926572, "Norm  Ampl"=-1.0311345636926572, "z∞ (V)"=-1.0311345636926572+0.0i, "4corners"={"z (-pi/2)"=-1.0311345636926572+0.5736824521422934i, "z(inf)"=-0.5200164984937075+1.0975277942502903i, "z (pi/2)"=-1.0311345636926572+0.5736824521422934i, "z center"=-0.5136528600391839+0.580046090596817i, "z(0)"=-0.5200164984937075+1.0975277942502903i, "radius"=-1.0311345636926572}}  # lorentzian
  n1 = control-ref of="cursor bracket in"() -> ()  [unwired: 1 out]
  n2 = Build Array("find fit action") -> (w15:T8[])
  n3 = Current VI's Path() -> ()  [unwired: 1 out]
  n4 = while {
    shift-right: [w46] -> _
    shift-left: w15 -> [w47]
    shift-right: [w31] -> w12
    shift-left: _ -> [w41]
    shift-right: [w36] -> w13
    shift-left: _ -> [w38]
    shift-right: [w35] -> _
    shift-left: _ -> [w40]
    shift-right: [w34] -> _
    shift-left: _ -> [w39]
    shift-right: [w37] -> w14
    shift-left: _ -> [w30]
    shift-right: [w32] -> w11
    shift-left: _ -> [w33]
    shift-right: [w28] -> w10
    shift-left: _ -> [w29]
    tunnel: "input" -> [w27]
    tunnel: "cursor bracket: fragment  ref" -> [w26]
    tunnel: "single fit parameters" -> [w25]
    tunnel: "omega map parameters" -> [w24]
    tunnel: "parameters: wavepacket" -> [w23]
    shift-right: [w21] -> _
    shift-left: _ -> [w22]
    tunnel: w4 -> [w20]
    tunnel: "plots: filter related" -> [w19]
    tunnel: "parameters: complex fit" -> [w18]
    tunnel: "plot what" -> [w17]
    stop <- w43 stop-if-true
    n5 = call "find peak action stack.vi"("stack action"=stack_action_--_control."pop", "command stack"=w47) -> ("find fit action out"=w42:T8, "command stack out"=w48:T8[])  [unwired: 7 in, 1 out]
    n6 = case shown="\"pm fit\"" w42 {
      tunnel: [w58 w62 w217 w368 w386 w404 w419 w459 w465 w487 w505 w523 w539 w568] -> w49
      tunnel: w48 -> [w58 w67 w222 w368 w386 w404 w419 w459 w465 w489 w507 w525 w539 w568]
      tunnel: w41 -> [w55 w66 w221 _ w375 w394 w411 w453 w470 _ _ _ w532 _]
      tunnel: w40 -> [w53 w70 w225 w364 w384 w402 w417 w450 w467 w483 w501 w519 _ w565]
      tunnel: w39 -> [w52 w69 w224 w363 w383 w401 w416 w449 w466 w482 w500 w518 _ w564]
      tunnel: w38 -> [w56 w63 w218 w366 w373 w392 w405 w452 w471 w484 w502 w520 w541 _]
      tunnel: [w57 w72 w227 w367 w385 w403 w418 w445 w464 w485 w503 w521 w528 w563] -> w37
      tunnel: [w56 w61 w216 w366 w372 w391 w409 w451 w469 w484 w502 w520 w541 w546] -> w36
      tunnel: [w53 w70 w225 w364 w384 w402 w417 w450 w467 w483 w501 w519 w536 w565] -> w35
      tunnel: [w52 w69 w224 w363 w383 w401 w416 w449 w466 w482 w500 w518 w535 w564] -> w34
      tunnel: w33 -> [w54 w71 w226 w365 w377 w396 w413 w430 w473 _ _ _ w540 w569]
      tunnel: [w54 w71 w226 w365 w376 w395 w412 w430 w472 w480 w498 w516 w540 w569] -> w32
      tunnel: [w55 w59 w214 w359 w374 w393 w410 w448 w468 w481 w499 w517 w532 w549] -> w31
      tunnel: w30 -> [w57 w72 w227 w367 w385 w403 w418 _ w464 w485 w503 w521 _ w563]
      tunnel: w29 -> [w51 w68 w223 _ w382 w400 w415 w429 w463 _ _ _ w533 w566]
      tunnel: [w51 w68 w223 w360 w382 w400 w415 w429 w463 w479 w497 w515 w534 w566] -> w28
      tunnel: w27 -> [_ _ _ _ w378 w390 _ _ _ _ _ _ _ _]
      tunnel: w26 -> [_ _ _ _ _ _ _ _ _ w476 w492 w510 _ _]
      tunnel: w25 -> [_ _ _ w359 _ _ _ _ _ w481 w499 w517 _ w549]
      tunnel: w24 -> [_ _ _ _ _ _ _ _ _ w480 w498 w516 _ _]
      tunnel: w23 -> [_ _ _ w360 _ _ _ _ _ w479 w497 w515 _ _]
      tunnel: w22 -> [w50 w64 w219 w358 w370 w387 w406 w447 w461 _ w495 w513 w530 w567]
      tunnel: [w50 w60 w215 w358 w370 w387 w406 w447 w461 w477 w493 w511 w530 w567] -> w21
      tunnel: w20 -> [_ _ _ _ _ _ _ _ _ w475 _ _ _ _]
      tunnel: w19 -> [_ _ _ _ _ _ _ _ _ _ _ _ _ w550]
      tunnel: w18 -> [_ _ _ _ _ _ _ _ _ _ _ _ _ w542]
      tunnel: w17 -> [_ _ _ _ _ _ _ _ _ _ _ _ _ w543]
      frame "empty", Default {
      }
      frame "-shake it one" {
        n7 = for {
          N: 1 -> [_]
          shift-right: [w93] -> _
          shift-left: _ -> [w91]
          shift-right: [w92] -> _
          shift-left: _ -> [w90]
          shift-right: [w87] -> w62
          shift-left: w67 -> [w95]
          shift-right: [w86] -> w61
          shift-left: w63 -> [w88]
          shift-right: [w85] -> w60
          shift-left: w64 -> [w89]
          shift-right: [w84] -> w59
          shift-left: w66 -> [w94]
          shift-right: [w76] -> _
          shift-left: _ -> [w74]
          shift-right: [w75] -> _
          shift-left: _ -> [w73]
          n8 = Unbundle By Name(w89) -> ("fancy fit.shakeit counter"=w81:i32)
          n9 = call "Q -- check range -- i -- integer.vi"("upper"="averaging -- # points", "lower"=1, "number"=w81) -> ("selector"=w82:T15)  [unwired: 6 in, 2 out]
          n10 = Divide(x="averaging -- span", y="averaging -- # points") -> (x/y=w77:dbl)
          n11 = case shown="\"above\", Default" w82 {
            tunnel: w95 -> [w110 w164 w201]
            tunnel: [w109 w163 w200] -> w87
            tunnel: w94 -> [w121 w147 w192]
            tunnel: [w124 w159 w195] -> w84
            tunnel: [w123 w142 w193] -> w93
            tunnel: [w122 w158 w194] -> w92
            tunnel: w91 -> [w123 _ w193]
            tunnel: w90 -> [w122 _ w194]
            tunnel: w89 -> [w114 w153 w189]
            tunnel: [w114 w152 w190] -> w85
            tunnel: w88 -> [w116 w145 w186]
            tunnel: [w115 w145 w186] -> w86
            tunnel: w77 -> [_ w130 w184]
            tunnel: w81 -> [w112 w139 w183]
            tunnel: "averaging -- # points" -> [_ w128 _]
            tunnel: "averaging -- win" -> [_ w131 _]
            tunnel: [w101 w127 w167] -> w76
            tunnel: [w100 0 w172] -> w75
            tunnel: w74 -> [w101 _ w169]
            tunnel: w73 -> [w100 _ w173]
            frame "above", Default {
              w107 = T8[] [enum."-find center"] items=["empty", "-find center", "-mapping", "fit", "-shake it one", "bbb", "-update pond", "move z(center)", "move z(inf)", "update pond", "fancy fit one", "fragment window moves", "-shake it two", "fancy fit two", "pm fit"]
              n12 = Unbundle By Name(w114) -> ("fancy fit.omega ave"=w118:dbl, "fancy fit.gamma ave"=w117:dbl, "fancy fit.window"=w120:dbl, "fancy fit.center"=w113:dbl, "cursor bracket: fragment  ref"=w119:refnum<vi>)
              n13 = Decrement(x=w112) -> (x-1=w111:i32)
              n14 = Divide(x=w117, y=w111) -> ()  [unwired: 1 out]
              n15 = Divide(x=w118, y=w111) -> ()  [unwired: 1 out]
              n16 = call "cursor window logic V2.vi"("cursor window action"=cursor_window_action."change cen&win", "window"=w120, "center"=w113, "cursor window in"=w119) -> ()  [unwired: 6 in, 2 out]
              n17 = call "find peak action stack.vi"("stack action"=stack_action_--_control."push", "find peak action list"=w107, "command stack"=w110) -> ("command stack out"=w109:T8[])  [unwired: 6 in, 2 out]
              n18 = Array Subset(array=w101, index=0, length=w100) -> (w105:cdb[])
              n19 = call "linear interpolation - bb - complex.vi"("Array"=w105) -> ("bb"=→"bb":dbl, "directed sigma"=→"directed sigma":dbl, "left"=→"left":cdb, "center"=w104:cdb, "right"=→"right":cdb)  [unwired: 6 in, 4 out]
              n20 = Bundle By Name(cluster=w121, "omega in window"=w123, "z in window"=w122) -> (w124:T11)
              n21 = Complex To Re/Im(x + iy=w104) -> (x=w103:dbl, y=w102:dbl)
              n22 = Bundle By Name(cluster=w116, "ω (Hz)"=w103, "Γ (Hz)"=w102) -> (w115:T1)
              "Numeric" <- w100
            }
            frame "below" {
              (unwired) 0.0
              w146 = 0.0 ("y")
              w165 = T8[] [enum."-find center", enum."-mapping", enum."-shake it one"] items=["empty", "-find center", "-mapping", "fit", "-shake it one", "bbb", "-update pond", "move z(center)", "move z(inf)", "update pond", "fancy fit one", "fragment window moves", "-shake it two", "fancy fit two", "pm fit"]
              n23 = Unbundle By Name(w147) -> ("omega in window"=w142:dbl[], "z in window"=w158:cdb[])
              n24 = Unbundle By Name(w153) -> ("cursor bracket: fragment  ref"=w150:refnum<vi>)
              n25 = property class="Clust (strict)"(reference=w150) -> (reference out=w143:refnum<vi>, "Value"=w151:T16)  [unwired: 1 in, 1 out]
              n26 = Unbundle By Name(w145) -> ("ω (Hz)"=w134:dbl)
              n27 = Array Max & Min(array=w142) -> (max value=w141:dbl, min value=w140:dbl)  [unwired: 2 out]
              n28 = Initialize Array(cdb 0.0+0.0i, w128) -> (w127:cdb[])
              n29 = Subtract(x=w141, y=w134) -> (x-y=w155:dbl)
              n30 = Subtract(x=w134, y=w140) -> (x-y=w156:dbl)
              n31 = Unbundle By Name(w151) -> ("center"=w149:dbl, "window"=w148:dbl)
              n32 = Max & Min(x=w155, y=w156) -> (min(x,y)=w157:dbl)  [unwired: 1 out]
              n33 = Multiply(x=w157, y=w131) -> (x*y=w137:dbl)
              n34 = Divide(x=w128, y=2.0) -> (x/y=w135:dbl)
              n35 = Multiply(x=w137, y=w130) -> (x*y=w136:dbl)
              n36 = Multiply(x=w136, y=w135) -> (x*y=w133:dbl)
              n37 = Increment(x=w139) -> (x+1=w154:i32)
              n38 = Subtract(x=w134, y=w133) -> (x-y=w132:dbl)
              n39 = call "find peak action stack.vi"("stack action"=stack_action_--_control."push", "find peak action list"=w165, "command stack"=w164) -> ("command stack out"=w163:T8[])  [unwired: 6 in, 2 out]
              n40 = call "cursor window logic V2.vi"("cursor window action"=cursor_window_action."change cen&win", "window"=w137, "center"=w132, "cursor window in"=w143) -> ("cursor window out"=w144:T9)  [unwired: 6 in, 1 out]
              n41 = call "acquire cursor window data.vi"("z in"=w158, "omega in"=w142, "cursor window"=w144) -> ("z out"=w160:cdb[], "omega  out"=w161:dbl[])  [unwired: 4 in, 3 out]
              n42 = Bundle By Name(cluster=w153, "fancy fit.omega ave"=w146, "fancy fit.gamma ave"=w146, "fancy fit.shakeit counter"=w154, "fancy fit.window"=w148, "fancy fit.center"=w149, "fancy fit.current window"=w137, "fancy fit.current center"=w132) -> (w152:T12)
              n43 = Bundle By Name(cluster=w147, "omega in window"=w161, "z in window"=w160) -> (w159:T11)
            }
            frame "in range" {
              w202 = T8[] [enum."-find center", enum."-mapping", enum."-shake it one"] items=["empty", "-find center", "-mapping", "fit", "-shake it one", "bbb", "-update pond", "move z(center)", "move z(inf)", "update pond", "fancy fit one", "fragment window moves", "-shake it two", "fancy fit two", "pm fit"]
              n44 = Unbundle By Name(w189) -> ("cursor bracket: fragment  ref"=w191:refnum<vi>, "fancy fit.current window"=w182:dbl, "fancy fit.current center"=w178:dbl)
              n45 = Unbundle By Name(w186) -> ("ω (Hz)"=w171:dbl, "Γ (Hz)"=w170:dbl)
              n46 = Multiply(x=w182, y=0.3 ("x")) -> (x*y=w179:dbl)
              n47 = Subtract(x=w178, y=w179) -> (x-y=w177:dbl)
              n48 = Add(x=w178, y=w179) -> (x+y=w180:dbl)
              n49 = call "Q - not nan -- real.vi"("Numeric"=w170) -> ("Boolean"=w175:bool)  [unwired: 9 in, 1 out]
              n50 = call "Q -- check range -- i -- real.vi"("upper"=w180, "lower"=w177, "number"=w171) -> ("in range?"=w176:bool)  [unwired: 6 in, 2 out]
              n51 = And(x=w175, y=w176) -> (x .and. y?=w174:bool)
              n52 = Re/Im To Complex(1:w170, 2:w171) -> (0:w168:cdb)
              n53 = case shown="True" w174 {
                tunnel: w173 -> [w204 w213]
                tunnel: [w204 w212] -> w172
                tunnel: w169 -> [w205 w209]
                tunnel: w168 -> [_ w207]
                tunnel: [w205 w206] -> w167
                frame False {
                }
                frame True {
                  n54 = Rotate 1D Array(1:w209, 2:1) -> (0:w210:cdb[])
                  n55 = Increment(x=w213) -> (x+1=w212:i32)
                  n56 = Replace Array Subset(array=w210, new element=w207, index=0) -> (w206:cdb[])
                }
              }
              n57 = Multiply(x=w184, y=w182) -> (x*y=w199:dbl)
              n58 = Increment(x=w183) -> (x+1=w188:i32)
              n59 = Add(x=w199, y=w178) -> (x+y=w187:dbl)
              n60 = call "cursor window logic V2.vi"("cursor window action"=cursor_window_action."change cen&win", "window"=w182, "center"=w187, "cursor window in"=w191) -> ("cursor window out"=w185:T9)  [unwired: 6 in, 1 out]
              n61 = call "acquire cursor window data.vi"("z in"=w194, "omega in"=w193, "cursor window"=w185) -> ("z out"=w196:cdb[], "omega  out"=w197:dbl[])  [unwired: 4 in, 3 out]
              n62 = call "find peak action stack.vi"("stack action"=stack_action_--_control."push", "find peak action list"=w202, "command stack"=w201) -> ("command stack out"=w200:T8[])  [unwired: 6 in, 2 out]
              n63 = Bundle By Name(cluster=w189, "fancy fit.shakeit counter"=w188, "fancy fit.current window"=w182, "fancy fit.current center"=w187) -> (w190:T12)
              n64 = Bundle By Name(cluster=w192, "omega in window"=w197, "z in window"=w196) -> (w195:T11)
            }
          }
        }
      }
      frame "-shake it two" {
        n65 = for {
          N: 1 -> [_]
          shift-right: [w250] -> _
          shift-left: _ -> [w248]
          shift-right: [w249] -> _
          shift-left: _ -> [w247]
          shift-right: [w244] -> w217
          shift-left: w222 -> [w252]
          shift-right: [w243] -> w216
          shift-left: w218 -> [w245]
          shift-right: [w242] -> w215
          shift-left: w219 -> [w246]
          shift-right: [w241] -> w214
          shift-left: w221 -> [w251]
          shift-right: [w233] -> _
          shift-left: _ -> [w231]
          shift-right: [w232] -> _
          shift-left: _ -> [w230]
          n66 = Unbundle By Name(w246) -> ("fancy fit.shakeit counter"=w238:i32)
          n67 = call "Q -- check range -- i -- integer.vi"("upper"="averaging -- # points 2", "lower"=1, "number"=w238) -> ("selector"=w239:T15)  [unwired: 6 in, 2 out]
          n68 = Divide(x="averaging -- span 2", y="averaging -- # points 2") -> (x/y=w234:dbl)
          n69 = case shown="\"in range\"" w239 {
            tunnel: w252 -> [w273 w308 w345]
            tunnel: [w272 w307 w344] -> w244
            tunnel: w251 -> [w277 w294 w337]
            tunnel: [w258 w303 w340] -> w241
            tunnel: [w279 w290 w338] -> w250
            tunnel: [w278 w302 w339] -> w249
            tunnel: w248 -> [w279 _ w338]
            tunnel: w247 -> [w278 _ w339]
            tunnel: w246 -> [w259 w300 w334]
            tunnel: [w259 w299 w335] -> w242
            tunnel: w245 -> [w255 w293 w332]
            tunnel: [w253 w293 w332] -> w243
            tunnel: w234 -> [_ _ _]
            tunnel: w238 -> [_ w289 w330]
            tunnel: "averaging -- # points 2" -> [_ w287 w314]
            tunnel: "averaging -- win 2" -> [_ _ _]
            tunnel: [w266 w286 w322] -> w233
            tunnel: [w265 0 w315] -> w232
            tunnel: w231 -> [w266 _ w324]
            tunnel: w230 -> [w265 _ w325]
            tunnel: "window factor - min" -> [_ w283 w318]
            tunnel: "window factor - max" -> [_ _ w317]
            frame "above", Default {
              w270 = T8[] [enum."-find center"] items=["empty", "-find center", "-mapping", "fit", "-shake it one", "bbb", "-update pond", "move z(center)", "move z(inf)", "update pond", "fancy fit one", "fragment window moves", "-shake it two", "fancy fit two", "pm fit"]
              n70 = Unbundle By Name(w259) -> ("fancy fit.window"=w276:dbl, "fancy fit.center"=w274:dbl, "cursor bracket: fragment  ref"=w275:refnum<vi>)
              n71 = call "find peak action stack.vi"("stack action"=stack_action_--_control."push", "find peak action list"=w270, "command stack"=w273) -> ("command stack out"=w272:T8[])  [unwired: 6 in, 2 out]
              n72 = Array Subset(array=w266, index=0, length=w265) -> (w268:cdb[])
              n73 = call "cursor window logic V2.vi"("cursor window action"=cursor_window_action."change cen&win", "window"=w276, "center"=w274, "cursor window in"=w275) -> ()  [unwired: 6 in, 2 out]
              n74 = call "linear interpolation - bb - complex.vi"("Array"=w268) -> ("bb"=→"bb 2":dbl, "directed sigma"=→"directed sigma 2":dbl, "left"=→"left 2":cdb, "center"=w267:cdb, "right"=→"right 2":cdb)  [unwired: 6 in, 4 out]
              n75 = Complex To Re/Im(x + iy=w267) -> (x=w256:dbl, y=w257:dbl)
              n76 = Bundle By Name(cluster=w277, "omega in window"=w279, "z in window"=w278) -> (w258:T11)
              n77 = Unbundle By Name(w255) -> ("4corners"=w254:T2)
              n78 = Unbundle By Name(w258) -> ("normalization factor"=w260:dbl)
              n79 = call "peak - calculate lorentzian.vi"("4corners"=w254, "normalization factor"=w260, "gamma"=w257, "omega"=w256) -> ("lorentzian out"=w253:T1)  [unwired: 7 in]
              "Numeric 2" <- w265
            }
            frame "below" {
              w309 = T8[] [enum."-find center", enum."-mapping", enum."-shake it two"] items=["empty", "-find center", "-mapping", "fit", "-shake it one", "bbb", "-update pond", "move z(center)", "move z(inf)", "update pond", "fancy fit one", "fragment window moves", "-shake it two", "fancy fit two", "pm fit"]
              n80 = Unbundle By Name(w294) -> ("omega in window"=w290:dbl[], "z in window"=w302:cdb[])
              n81 = Unbundle By Name(w300) -> ("cursor bracket: fragment  ref"=w297:refnum<vi>)
              n82 = property class="Clust (strict)"(reference=w297) -> (reference out=w291:refnum<vi>, "Value"=w298:T16)  [unwired: 1 in, 1 out]
              n83 = Unbundle By Name(w293) -> ("ω (Hz)"=w282:dbl, "Γ (Hz)"=w284:dbl)
              n84 = Initialize Array(cdb 0.0+0.0i, w287) -> (w286:cdb[])
              n85 = Unbundle By Name(w298) -> ("center"=w296:dbl, "window"=w295:dbl)
              n86 = Multiply(x=w284, y=w283) -> (x*y=w281:dbl)
              n87 = Increment(x=w289) -> (x+1=w301:i32)
              n88 = call "find peak action stack.vi"("stack action"=stack_action_--_control."push", "find peak action list"=w309, "command stack"=w308) -> ("command stack out"=w307:T8[])  [unwired: 6 in, 2 out]
              n89 = call "cursor window logic V2.vi"("cursor window action"=cursor_window_action."change cen&win", "window"=w281, "center"=w282, "cursor window in"=w291) -> ("cursor window out"=w292:T9)  [unwired: 6 in, 1 out]
              n90 = call "acquire cursor window data.vi"("z in"=w302, "omega in"=w290, "cursor window"=w292) -> ("z out"=w304:cdb[], "omega  out"=w305:dbl[])  [unwired: 4 in, 3 out]
              n91 = Bundle By Name(cluster=w300, "fancy fit.shakeit counter"=w301, "fancy fit.window"=w295, "fancy fit.center"=w296, "fancy fit.current center"=w282, "fancy fit.current window"=w281) -> (w299:T12)
              n92 = Bundle By Name(cluster=w294, "omega in window"=w305, "z in window"=w304) -> (w303:T11)
            }
            frame "in range" {
              w346 = T8[] [enum."-find center", enum."-mapping", enum."-shake it two"] items=["empty", "-find center", "-mapping", "fit", "-shake it one", "bbb", "-update pond", "move z(center)", "move z(inf)", "update pond", "fancy fit one", "fragment window moves", "-shake it two", "fancy fit two", "pm fit"]
              n93 = Unbundle By Name(w334) -> ("cursor bracket: fragment  ref"=w336:refnum<vi>, "fancy fit.current window"=w319:dbl, "fancy fit.current center"=w320:dbl)
              n94 = Unbundle By Name(w332) -> ("ω (Hz)"=w321:dbl, "Γ (Hz)"=w312:dbl)
              n95 = Multiply(x=w319, y=0.3 ("x")) -> ()  [unwired: 1 out]
              n96 = call "Q - not nan -- real.vi"("Numeric"=w312) -> ("Boolean"=w327:bool)  [unwired: 9 in, 1 out]
              n97 = call "Q -- check range -- i -- real - window.vi"("window"=w319, "center"=w320, "number"=w321) -> ("in range?"=w328:bool)  [unwired: 6 in, 2 out]
              n98 = And(x=w327, y=w328) -> (x .and. y?=w326:bool)
              n99 = Re/Im To Complex(1:w312, 2:w321) -> (0:w323:cdb)
              n100 = case shown="True" w326 {
                tunnel: w325 -> [w348 w357]
                tunnel: [w348 w356] -> w315
                tunnel: w324 -> [w349 w353]
                tunnel: w323 -> [_ w351]
                tunnel: [w349 w350] -> w322
                frame False {
                }
                frame True {
                  n101 = Rotate 1D Array(1:w353, 2:1) -> (0:w354:cdb[])
                  n102 = Increment(x=w357) -> (x+1=w356:i32)
                  n103 = Replace Array Subset(array=w354, new element=w351, index=0) -> (w350:cdb[])
                }
              }
              n104 = Divide(x=w315, y=w314) -> (x/y=w316:dbl)
              n105 = call "Q -- get  number in range.vi"("right"=w317, "left"=w318, "fraction"=w316) -> ("number in range"=w313:dbl)  [unwired: 8 in]
              n106 = Increment(x=w330) -> (x+1=w333:i32)
              n107 = Multiply(x=w312, y=w313) -> (x*y=w311:dbl)
              n108 = call "cursor window logic V2.vi"("cursor window action"=cursor_window_action."change cen&win", "window"=w311, "center"=w321, "cursor window in"=w336) -> ("cursor window out"=w331:T9)  [unwired: 6 in, 1 out]
              n109 = call "acquire cursor window data.vi"("z in"=w339, "omega in"=w338, "cursor window"=w331) -> ("z out"=w341:cdb[], "omega  out"=w342:dbl[])  [unwired: 4 in, 3 out]
              n110 = call "find peak action stack.vi"("stack action"=stack_action_--_control."push", "find peak action list"=w346, "command stack"=w345) -> ("command stack out"=w344:T8[])  [unwired: 6 in, 2 out]
              n111 = Bundle By Name(cluster=w334, "fancy fit.shakeit counter"=w333, "fancy fit.current center"=w321, "fancy fit.current window"=w311) -> (w335:T12)
              n112 = Bundle By Name(cluster=w337, "omega in window"=w342, "z in window"=w341) -> (w340:T11)
            }
          }
        }
      }
      frame "update pond" {
        w361 = T8[] [enum."-update pond"] items=["empty", "-find center", "-mapping", "fit", "-shake it one", "bbb", "-update pond", "move z(center)", "move z(inf)", "update pond", "fancy fit one", "fragment window moves", "-shake it two", "fancy fit two", "pm fit"]
        n113 = call "find peak action stack.vi"("stack action"=stack_action_--_control."push", "find peak action list"=w361) -> ()  [unwired: 7 in, 3 out]
      }
      frame "move z(center)" {
        w379 = T17."replace z(center) -- keepin z(inf) the same"  # action
        n114 = Unbundle By Name(w370) -> ("cursor bracket: fragment  ref"=w369:refnum<vi>)  [unwired: 1 out]
        n115 = property class="Clust (strict)"(reference=w369) -> ("Value"=w371:T16)  [unwired: 1 in, 2 out]
        n116 = call "move lorentzian.vi"("action"=w379, "new z(center)"=w378, "lorentzian in"=w373) -> ("lorentzian out"=w380:T1)  [unwired: 8 in]
        n117 = call "lorentzian from circle corners V7.vi"("cursor bracket in"=w371, "update z(inf)"=enum16{"update z(inf)", "do not update z(inf)"}."do not update z(inf)", "omega map rameters in"=w377, "parameters in: center detection"=w375, "lorentzian in"=w380) -> ("omega map parameters  out"=w376:T10, "parameters out  : center detection"=w374:T11, "lorentzian out"=w372:T1)  [unwired: 4 in]
      }
      frame "move z(inf)" {
        w397 = T17."replace z(inf)  -- keeping z(center) the same"  # action
        n118 = Unbundle By Name(w387) -> ("cursor bracket: fragment  ref"=w389:refnum<vi>)  [unwired: 1 out]
        n119 = call "move lorentzian.vi"("action"=w397, "new z(inf)"=w390, "lorentzian in"=w392) -> ("lorentzian out"=w398:T1)  [unwired: 8 in]
        n120 = property class="Clust (strict)"(reference=w389) -> ("Value"=w388:T16)  [unwired: 1 in, 2 out]
        n121 = call "lorentzian from circle corners V7.vi"("cursor bracket in"=w388, "update z(inf)"=enum16{"update z(inf)", "do not update z(inf)"}."do not update z(inf)", "omega map rameters in"=w396, "parameters in: center detection"=w394, "lorentzian in"=w398) -> ("omega map parameters  out"=w395:T10, "parameters out  : center detection"=w393:T11, "lorentzian out"=w391:T1)  [unwired: 4 in]
      }
      frame "fragment window moves" {
        n122 = Unbundle By Name(w406) -> ("cursor bracket: fragment  ref"=w408:refnum<vi>)  [unwired: 1 out]
        n123 = property class="Clust (strict)"(reference=w408) -> ("Value"=w407:T16)  [unwired: 1 in, 2 out]
        n124 = call "lorentzian from circle corners V7.vi"("cursor bracket in"=w407, "update z(inf)"=enum16{"update z(inf)", "do not update z(inf)"}."do not update z(inf)", "omega map rameters in"=w413, "parameters in: center detection"=w411, "lorentzian in"=w405) -> ("omega map parameters  out"=w412:T10, "parameters out  : center detection"=w410:T11, "lorentzian out"=w409:T1)  [unwired: 4 in]
      }
      frame "-find center" {
        # "(1) determine complex region"
        # "(3) generate interference\npattern to find center of the circle"
        # "(2) decimate to 2D grid"
        n125 = Unbundle By Name(w453) -> ("number of 2D grid points"=w431:i32, "z in window"=w458:cdb[], "pond scale factor"=w446:dbl, "decimation threshold"=w454:i32, "omega in window"=w437:dbl[], "dz/domega"=w436:cdb[])
        n126 = Unbundle By Name(w429) -> ("wave number"=w428:dbl, "delta k"=w427:dbl)
        n127 = call "find fit -- set up complex region - V2.vi"("scale factor"=w446) -> ("complex region"=w445:T7)  [unwired: 10 in]
        n128 = call "find fit -- normalize complex culture.vi"("z in window"=w458) -> ("z  normalized"=w455:cdb[], "normalization factor"=w456:dbl, "data center"=w457:cdb, "# of elements"=w442:i32)  [unwired: 7 in]
        n129 = call "peak -- get weights.vi"("dz/domega"=w436, "omega"=w437) -> ()  [unwired: 8 in, 2 out]
        n130 = call "smart decimate  - V2.vi"("number of 2D grid points"=w431, "complex region"=w445, "omega in"=w437, "decimation threshold"=w454, "z in"=w455) -> ("number of decimated elements"=w441:i32, "decimated omega"=w444:dbl[], "decimated z"=w434:cdb[])  [unwired: 4 in]
        n131 = Decrement(x=w441) -> (x-1=w440:i32)
        n132 = Index Array(array=w444, index #1=0 ("index"), index #2=w440) -> (element #1=w439:dbl, element #2=w438:dbl)
        n133 = Complex To Re/Im(x + iy=w434) -> (x=w433:dbl[], y=w432:dbl[])
        n134 = Array Size(array=w434) -> (size(s)=w435:i32)
        n135 = Bundle By Name(cluster=w453, "# of points in window"=w442, "# of points in pond"=w441, "normalization factor"=w456, "normalized z"=w455, "decimated omega"=w444, "decimated z"=w434, "data center"=w457, "min omega"=w439, "max omega"=w438) -> (w448:T11)
        n136 = dll-call lib="C:/Users/riggslab/Desktop/Arkady/maglab ultrasound -- arkady -- extended/circledll.dll" fn="?find_center_cashed@@YAHPAN0HHNN00PAH@Z"("re"=w433, "im"=w432, "nPoints"=w435, "nGrid"=w431, "wave_num"=w428, "decay"=w427, "center_re"=0.0, "center_im"=0.0, "counter_out"=1) -> ("center_re"=w424:dbl, "center_im"=w423:dbl, "counter_out"=→"counter_out":i32)  [unwired: 10 in, 2 out]
        n137 = Re/Im To Complex(1:w423, 2:w424) -> (0:w422:cdb)
        n138 = Bundle By Name(cluster=w452, "4corners.z center"=w422) -> (w451:T1)
      }
      frame "-mapping" {
        n139 = Unbundle By Name(w461) -> ("cursor bracket: fragment  ref"=w462:refnum<vi>)
        n140 = property class="Clust (strict)"(reference=w462) -> ("Value"=w460:T16)  [unwired: 1 in, 2 out]
        n141 = call "lorentzian from circle corners V7.vi"("cursor bracket in"=w460, "update z(inf)"=enum16{"update z(inf)", "do not update z(inf)"}."update z(inf)", "omega map rameters in"=w473, "parameters in: center detection"=w470, "lorentzian in"=w471) -> ("omega map parameters  out"=w472:T10, "parameters out  : center detection"=w468:T11, "lorentzian out"=w469:T1)  [unwired: 4 in]
      }
      frame "fit" {
        n142 = Bundle By Name(cluster=w475, "cursor bracket: fragment  ref"=w476) -> (w477:T12)
        n143 = Unbundle By Name(w479) -> ("wavepacket is"=w478:bool)
        n144 = case shown="True" w478 {
          tunnel: [w490 w491] -> w486
          frame True {
            w490 = T8[] [enum."-find center", enum."-mapping"] items=["empty", "-find center", "-mapping", "fit", "-shake it one", "bbb", "-update pond", "move z(center)", "move z(inf)", "update pond", "fancy fit one", "fragment window moves", "-shake it two", "fancy fit two", "pm fit"]
          }
          frame False {
            w491 = T8[] [enum."-update pond", enum."-find center", enum."-mapping"] items=["empty", "-find center", "-mapping", "fit", "-shake it one", "bbb", "-update pond", "move z(center)", "move z(inf)", "update pond", "fancy fit one", "fragment window moves", "-shake it two", "fancy fit two", "pm fit"]
          }
        }
        n145 = call "find peak action stack.vi"("stack action"=stack_action_--_control."push", "find peak action list"=w486, "command stack"=w489) -> ("command stack out"=w487:T8[])  [unwired: 6 in, 2 out]
      }
      frame "fancy fit one" {
        n146 = Unbundle By Name(w497) -> ("wavepacket is"=w496:bool)
        n147 = case shown="False" w496 {
          tunnel: [w508 w509] -> w504
          frame True {
            w508 = T8[] [enum."-find center", enum."-mapping", enum."-shake it one"] items=["empty", "-find center", "-mapping", "fit", "-shake it one", "bbb", "-update pond", "move z(center)", "move z(inf)", "update pond", "fancy fit one", "fragment window moves", "-shake it two", "fancy fit two", "pm fit"]
          }
          frame False {
            w509 = T8[] [enum."-update pond", enum."-find center", enum."-mapping", enum."-shake it one"] items=["empty", "-find center", "-mapping", "fit", "-shake it one", "bbb", "-update pond", "move z(center)", "move z(inf)", "update pond", "fancy fit one", "fragment window moves", "-shake it two", "fancy fit two", "pm fit"]
          }
        }
        n148 = Bundle By Name(cluster=w495, "cursor bracket: fragment  ref"=w492, "fancy fit.shakeit counter"=0) -> (w493:T12)
        n149 = call "find peak action stack.vi"("stack action"=stack_action_--_control."push", "find peak action list"=w504, "command stack"=w507) -> ("command stack out"=w505:T8[])  [unwired: 6 in, 2 out]
      }
      frame "fancy fit two" {
        n150 = Unbundle By Name(w515) -> ("wavepacket is"=w514:bool)
        n151 = case shown="True" w514 {
          tunnel: [w526 w527] -> w522
          frame True {
            w526 = T8[] [enum."-find center", enum."-mapping", enum."-shake it two"] items=["empty", "-find center", "-mapping", "fit", "-shake it one", "bbb", "-update pond", "move z(center)", "move z(inf)", "update pond", "fancy fit one", "fragment window moves", "-shake it two", "fancy fit two", "pm fit"]
          }
          frame False {
            w527 = T8[] [enum."-update pond", enum."-find center", enum."-mapping", enum."-shake it two"] items=["empty", "-find center", "-mapping", "fit", "-shake it one", "bbb", "-update pond", "move z(center)", "move z(inf)", "update pond", "fancy fit one", "fragment window moves", "-shake it two", "fancy fit two", "pm fit"]
          }
        }
        n152 = Bundle By Name(cluster=w513, "cursor bracket: fragment  ref"=w510, "fancy fit.shakeit counter"=0) -> (w511:T12)
        n153 = call "find peak action stack.vi"("stack action"=stack_action_--_control."push", "find peak action list"=w522, "command stack"=w525) -> ("command stack out"=w523:T8[])  [unwired: 6 in, 2 out]
      }
      frame "-update pond" {
        n154 = Unbundle By Name(w532) -> ("number of 2D grid points"=w531:i32, "pond scale factor"=w529:dbl)
        n155 = call "find fit -- set up complex region - V2.vi"("scale factor"=w529) -> ("complex region"=w528:T7)  [unwired: 10 in]
        n156 = call "generate wave packet V2.vi"("number of grid points"=w531, "complex region"=w528, "wavepacket in"=w533) -> ("pond array out"=w535:cdb[][], "wavepacket array out"=w536:cdb[][], "wavepacket out"=w537:T4)  [unwired: 6 in]
        n157 = Bundle By Name(cluster=w537, "wavepacket is"=TRUE) -> (w534:T4)
      }
      frame "pm fit" {
        n158 = Unbundle By Name(w549) -> ("omega in window"=w548:dbl[], "z in window"=w547:cdb[])
        n159 = Unbundle By Name(w542) -> ("span"=w553:dbl)
        n160 = call "filter - complex - four.vi"("omega (Hz) in"=w548, "z in"=w547, "span"=w553) -> ("center"=w559:cdb, "norm"=w558:dbl, "omega out"=w560:dbl[], "z in out"=w561:cdb[], "z out"=w554:cdb[], "win omega out"=w557:dbl[], "dz/domega out"=w556:cdb[], "tale of three"=w562:T18)  [unwired: 9 in]
        n161 = call "peak -- PM find lorenzian - V2.vi"("omega"=w560, "z"=w554, "dz/domega"=w556) -> ("phase (around center)"=w555:dbl[], "weights"=w545:dbl[], "cp lorentzian"=w551:T1, "poor man lorentzian"=w546:T1)  [unwired: 9 in]
        "pm lorentzian" <- w546
        "cp lorentzian" <- w551
        "good lorentzian" <- w546
        n162 = case shown="\"plot cp\"" enum16{"plot pm", "plot cp", "a"}."plot pm" ("plot what") {
          tunnel: [w582 w583] -> w544
          tunnel: w551 -> [_ w583]
          tunnel: w546 -> [w582 _]
          frame "plot pm", Default {
          }
          frame "plot cp" {
          }
        }
        n163 = case shown="\"dont plot\"" w543 {
          tunnel: w562 -> [w581 _]
          tunnel: w561 -> [w580 _]
          tunnel: w560 -> [w579 _]
          tunnel: w559 -> [w578 _]
          tunnel: w558 -> [w577 _]
          tunnel: w557 -> [w576 _]
          tunnel: w555 -> [w575 _]
          tunnel: w554 -> [w574 _]
          tunnel: w550 -> [w573 _]
          tunnel: w542 -> [w572 _]
          tunnel: w545 -> [w571 _]
          tunnel: w544 -> [w570 _]
          frame "plot", Default {
            n164 = call "filter pipe - plot staff - more - V2.vi"("omega  in"=w579, "zin"=w580, "z out"=w574, "win omega"=w576, "phase"=w575, "dz/domega in"=w571, "center"=w578, "plots: filter related"=w573, "norm"=w577, "parameters: complex fit"=w572, "tale of three indices -- int -- control"=w581, "lorentzian"=w570) -> ()  [unwired: 8 in]
          }
          frame "dont plot" {
          }
        }
      }
    }
    n165 = call "find peak action stack.vi"("stack action"=stack_action_--_control."check", "command stack"=w49) -> ("stack is empty ?"=w43:bool, "command stack out"=w46:T8[])  [unwired: 7 in, 1 out]
  }
  "lorentzian out" <- w13
  "single fit parameters out" <- w12
  "omega map parameters out" <- w11
  "complex region out" <- w14
  "parameters: wavepacket  out" <- w10
